vi "Old_XLIN1.7-2048SQ TE0_Host.vi"() -> ()   [LabVIEW 2018]
uses:
  <instrlib>/niDCPower/nidcpower.llb/niDCPower Measurement Type.ctl
  <instrlib>/niDMM/nidmm.llb/niDMM Function.ctl
  <instrlib>/niDMM/nidmm.llb/niDMM Resolution in Digits.ctl
  <vilib>/FPGAPlugInAG/PXI-7953R/niLvFpga_Open_PXI-7953R.vi
  <vilib>/rvi/interface/common/dynamic/niFpgaDynamicAddResources.vi
  <vilib>/FPGAPlugInAG/Dynamic/niLvFpga_Reset_Dynamic.vi
  <vilib>/FPGAPlugInAG/Dynamic/niLvFpga_Run_Dynamic.vi
  <vilib>/Utility/error.llb/Error Cluster From Error Code.vi
  <vilib>/rvi/errors/niLvFpgaAdjustHostInterfaceError.vi
  <instrlib>/niDMM/nidmm.llb/niDMM Configure Measurement Digits.vi
  <vilib>/FPGAPlugInAG/Dynamic/niLvFpga_Close_Dynamic.vi
  <vilib>/rvi/interface/nirviOpenFPGA/nirviOpenFPGA.xnode
  FPGA Bitfiles/XLIN1.7-2048SQTE_FPGATarget_XLIN1.7-2048SQTE_AuhCl0rpp4A.lvbitx
  <vilib>/rvi/interface/nirviMethod/nirviMethod.xnode
  <vilib>/rvi/interface/nirviReadWriteControl/nirviReadWriteControl.xnode
  <vilib>/rvi/interface/nirviCloseFPGA/nirviCloseFPGA.xnode
  NiFpgaLv.dll
  <vilib>/rvi/interface/Simulation/niFpgaSimulationCallBeginRW.vi
  <vilib>/FPGAPlugInAG/Dynamic/niLvFpga_ReadFifo_Dynamic.vi
  <vilib>/rvi/errors/niLvFpgaMergeErrorWithErrorCode.vi
panel:
  in  "Tab Control":T1(tab)
  in  "Clean Table":bool caption="Clear"
  in  "VDDD ON":bool
  out "VDDD_char":dbl(graph)=8.200132019086688e-05
  in  "VDDD, V":dbl=3.3000000000000003 caption="voltage level" min=0.0 max=6.0 format="%_6p"
  out "VDDD_cur, A":dbl=8.200132019086688e-05 caption="measurement" format="%_6g"
  in  "VDDD_curlim, A":dbl=0.5 caption="current limit" min=0.01 max=1.0 format="%_6p"
  in  "VDDD_selcur, A":dbl=0.49 caption="current limit" format="%_6p"
  out "VDDA_warning":bool caption="VCC_warning"
  out "VDDD_counter":u32 caption="VCC_counter"
  in  "VDDA ON":bool
  out "VDDA_char":dbl(graph)=9.464711192498274e-07
  in  "VDDA, V":dbl=3.3 caption="voltage level" min=0.0 max=20.0 format="%_6p"
  out "VDDA_cur, A":dbl=9.464711192498274e-07 caption="measurement" format="%_6g"
  in  "VDDA_curlim, A":dbl=0.5 caption="current limit" min=0.01 max=1.0 format="%_6p"
  in  "VDDA_selcur, A":dbl=0.49 caption="current limit" format="%_6p"
  out "VDDD_warning":bool caption="VCC_warning"
  out "VDDA_counter":u32 caption="VCC_counter"
  in  "Logs Path":path=path "D:/NI LabVIEW/21.056 XLIN1.7-2048SQ TE0/LOGS"
  in  "DC POWER 1":refnum<k15>="PXI1Slot2_2" caption="VСС_+5"
  in  "DC POWER 2":refnum<k15>="PXI1Slot3_3" caption="VСС_+5"
  in  "FPGA":tag="RIO0"
  in  "LED IR ON":bool
  out "LED IR_char":dbl(graph)=1.4003158139382402e-06
  in  "LED IR, V":dbl=-1.3000000000000003 caption="voltage level" min=-20.0 max=0.0 format="%_6p"
  out "LED IR_cur, A":dbl=1.4003158139382402e-06 caption="measurement" format="%_6g"
  in  "LED IR_curlim, A":dbl=0.4 caption="current limit" min=0.01 max=1.0 format="%_6p"
  out "Образец №":string
  in  "STOP":bool
  out "FIFOIsDone":bool
  out "FirmwareIsDone":bool
  out "PreCaptureIsDone":bool
  out "Frame Is Done":bool
  in  "Save":bool
  in  "Темный(F)\nСветлый(T)":bool
  in  "Примечание":string
  in  "VDDA_Clear_SEL":bool caption="Clear"
  in  "VDDD_Clear_SEL":bool caption="Clear"
  in  "Capture":bool
  in  "SEL Poll Time":u32=1
  in  "Автомат":bool
  in  "Питание":bool
  in  "SIM_SEL":bool
  in  "Loop Capture":bool
  in  "NI DMM":refnum<k15>="PXI1Slot4"
  in  "Опросить DMM":bool caption="Опрос DMM"
  in  "U_AOS Table":string[][](table)=[["", "Voltage", "", ""], ["OutTop_n", "", "", ""], ["OutTop_p", "", "", ""], ["OutBot_p", "", "", ""], ["OutBot_n", "", "", ""], ["U_AOS_Top", "", "", ""], ["U_AOS_Bot", "", "", ""]] caption="Размах аналогового выхода"
  in  "RS":bool
  in  "Очистить ОС":bool caption="Clear"
  out "Счетчик ОС":u32
  in  "+0.5_Clear_SEL":bool caption="Clear"
  out "+6_counter":u32 caption="VCC_counter"
  out "+6_warning":bool caption="VCC_warning"
  in  "+6_selcur, A":dbl=0.49 caption="current limit" format="%_6p"
  in  "+6, A":dbl=0.5 caption="current limit" min=0.01 max=1.0 format="%_6p"
  out "+6_cur, A":dbl=0.00011627237241327378 caption="measurement" format="%_6g"
  in  "+6, V":dbl=6.0 caption="voltage level" min=0.0 max=6.0 format="%_6p"
  out "+6_char":dbl(graph)=0.00011627237241327378
  in  "+6 ON":bool
  in  "Этап прошивки":T2(ring)
  in  "Firmware":bool
  out "Command":u8[](array[numeric])
  out "Data":u8[](array[numeric])
  out "ArraySize":u8
  in  "XLIN Rise Time":u32=500
  out "ADC Configuration":bool
  in  "Frame Poll Time":u32=500
  out "+0.5_counter":u32 caption="VCC_counter"
  out "+0.5_warning":bool caption="VCC_warning"
  in  "+0.5_selcur, A":dbl=0.09 caption="current limit" format="%_6p"
  in  "+0.5_curlim, A":dbl=0.1 caption="current limit" min=0.01 max=1.0 format="%_6p"
  out "+0.5_cur, A":dbl=-6.586231837824974e-06 caption="measurement" format="%_6g"
  in  "+0.5, V":dbl=0.5 caption="voltage level" min=0.0 max=20.0 format="%_6p"
  out "+0,5_char":dbl(graph)=-6.586231837824974e-06
  in  "+0.5 ON":bool
  in  "ОС":bool
  out "Счетчик ФС":u32
  in  "Очистить ФС":bool caption="Clear"
  in  "Минус ОС":bool
  in  "Плюс ОС":bool
  in  "Минус ФС":bool
  in  "Плюс ФС":bool
  in  "ADC Rise Time":u32=500
  out "АЦП прошит!":bool
  in  "ФС":bool
  in  "Задержка прошивки":u32=1
  out "Power VDDD+VDDA, mW":string
  in  "+6_Clear_SEL":bool caption="Clear"
  out "Image":T3(plugin-control)
  in  "Top":bool=TRUE
  in  "Bot":bool=TRUE
  in  "Capture Format":enum16{"Top / Bot", "Top & Bot"}(ring)
  in  "Frame Exposure, ms":u32=100
  in  "Delay Between Top&Bot":u32=5
  out "Configuration":bool[](array[boolean])
  in  "3CH/1CH":enum16{"3CH", "1CH"}(ring)=enum."1CH"
  in  "2/4 V":enum16{"2V", "4V"}(ring)=enum."4V"
  in  "+/- GREEN":enum16{"-", "+"}(ring)=enum."+"
  in  "Смещение, до 300_GREEN":dbl
  in  "+/- RED":enum16{"-", "+"}(ring)=enum."+"
  in  "Смещение, до 300_RED":dbl
  in  "+/- BLUE":enum16{"-", "+"}(ring)=enum."+"
  in  "Смещение, до 300_BLUE":dbl
  in  "Усиление (до 6)_GREEN":u8=1
  in  "Усиление (до 6)_BLUE":u8=1
  in  "Усиление (до 6)_RED":u8=1
  in  "Какой канал?":enum16{"GREEN", "RED", "BLUE"}(ring)=enum."BLUE"
  in  "Прошить АЦП":bool
  in  "ADC Register Map":T4(ring)
  out "MUX":bool[](array[boolean])
  in  "TopVIN":enum16{"GREEN", "RED", "BLUE"}(ring)=enum."RED"
  in  "Bot VIN":enum16{"GREEN", "RED", "BLUE"}(ring)
  in  "7..0(F)/0..7(T)":bool
  in  "F(F)/R(T)_CmAD":bool
  in  "F(F)/R(T)_FIFO":bool=TRUE
  in  "Command CS":u8[](array[numeric])=[8, 4, 2, 2, 2, 2, 2, 2, 2, 2, 2, 2, 2, 2, 2, 2, 2, 2, 2, 2, 2, 2, 2, 2, 2, 2, 2, 2, 2, 2, 2, 2, 2, 8, 4, 1, 1, 1, 1, 1, 1, 1, 1, 1, 0]
  in  "Data CSTop":u8[](array[numeric])=[0, 9, 12, 11, 0, 6, 0, 2, 11, 0, 8, 0, 0, 0, 0, 9, 1, 3, 3, 7, 15, 15, 5, 15, 0, 1, 15, 15, 5, 8, 5, 2, 3, 0, 8, 2, 3, 3, 3, 3, 3, 3, 3, 2, 0]
  in  "Data CSBot":u8[](array[numeric])=[0, 9, 8, 11, 0, 6, 0, 2, 11, 0, 8, 0, 0, 0, 0, 9, 1, 3, 11, 7, 15, 15, 5, 15, 0, 1, 15, 15, 5, 8, 5, 2, 3, 0, 8, 2, 3, 3, 3, 3, 3, 3, 3, 2, 0]
  in  "Command Reset":u8[](array[numeric])=[8, 4, 2, 2, 2, 2, 9, 0]
  in  "Data Reset":u8[](array[numeric])=[0, 0, 0, 5, 0, 0, 0, 0]
  in  "Command Hold":u8[](array[numeric])=[8, 4, 2, 2, 2, 2, 9, 2, 2, 2, 2, 2, 0, 0, 0, 0, 0, 8, 4, 2, 2, 2, 2, 9, 2, 2, 2, 2, 9, 2, 2, 2, 2, 9, 2, 2, 2, 2, 9, 2, 2, 2, 2, 9, 2, 2, 2, 2, 9, 0, 0]
  in  "Data Hold":u8[](array[numeric])=[0, 0, 0, 1, 1, 0, 0, 0, 5, 1, 0, 0, 0, 0, 0, 0, 0, 0, 0, 0, 3, 1, 0, 0, 1, 5, 1, 0, 0, 1, 3, 1, 0, 0, 1, 3, 1, 0, 0, 1, 11, 1, 11, 0, 1, 11, 1, 3, 0, 0, 0]
  in  "Command Sample Start":u8[](array[numeric])=[8, 4, 2, 2, 2, 2, 9, 2, 2, 2, 2, 2, 2, 1, 1, 1, 1, 1, 1, 0]
  in  "Data Sample Start":u8[](array[numeric])=[0, 0, 1, 11, 1, 0, 0, 0, 0, 6, 0, 0, 15, 0, 1, 3, 5, 13, 13, 0]
  in  "Command Sample End":u8[](array[numeric])=[8, 4, 2, 0, 0]
  in  "Data Sample End":u8[](array[numeric])=[0, 5, 1, 0, 0]
  in  "Supply Select":u8(ring) items=["Local", "External"]
  in  "1032 pixels":u16=1032
  in  "NumberOfAddFIFO":u16=2064
  in  "Falling CLK_1 = 1":u8=1
  in  "Rising CLK_1 = 0":u8
  in  "Rising CLK_2 = 1":u8=1
  in  "Falling CLK_2 = 2":u8=2
  in  "Rising CLK_3 = 1":u8=1
  in  "Falling CLK_3 = 1":u8=1
  in  "Falling CLK_4 = 3":u8=3
  in  "Rising CLK_4 = 2":u8=2
  in  "Rising CLK_5 = 2":u8=2
  in  "Falling CLK_5 = 2":u8=2
  in  "Falling CLK_6 = 2":u8=2
  in  "Rising CLK_6 = 2":u8=1
  in  "Falling CLK_7 = 1":u8=1
  in  "Rising CLK_7 = 1":u8=1
  in  "Counter R&F CLK_1 = 7":u8=7
  in  "Counter R&F CLK_2 = 4":u8=4
  in  "R ADCCLK = 5":u16=5
  in  "R MCLK = 2":u16=2
  in  "Counter R CLK = 2":u8=2
  out "FIFOCounter":u16
  out "SEL output file refnum":refnum<file>
  out "Power OFF":bool
  in  "Считать SIM SEL":bool
  out "Ready Status":bool
  out "NI DMM Real Voltage":dbl format="%.15f"
  out "NI DMM output file":refnum<file>
  out "NI DMM Voltage":dbl caption="Voltage" format="%_6g"
  out "NI DMM Voltage Char":dbl(graph)=0.6705812438667635
  in  "NI DMM units":string(combo)="1" caption="Units"
  in  "NI DMM Voltage Range":string(combo)="10" caption="Range"
  in  "NI DMM Poll Time":u32=100 caption="DMM Poll Time"
  in  "NI DMM Samples":i32=10
  out "Voltage Sum":dbl format="%.15f"
  in  "U_AOS":dbl[](array[numeric])=[0.0, 0.0, 0.0, 0.0, 0.0, 0.0]
  in  "PreCapture":bool
  in  "Start":bool
  out "SEL_warning":bool caption="SEL"
  out "Test Model Log Path":path
  out "Bot Pixel":bool[](array[boolean])
  out "Top Pixel":bool[](array[boolean])
  out "FrameDataFromTop":u8[](array[numeric])
  out "FrameDataFromBot":u8[](array[numeric])
  out "LineOfBot":u16[](array[numeric])
  out "LineOfTop":u16[](array[numeric])
  in  "WatchDogFIFOTime":u32=1000
  out "FIFOTime":u32
  out "Full Line":u16[](array[numeric])
  # "CH0 VDDD\nCH1 VDDA\nCH2 LED IR"
  # "CH0 +6\nCH1 +0,5"
  # "DC1 CH0"
  # "DC1 CH1"
  # "DC2 CH1"
  # "DC2 CH2"
  # "DC2 CH2"
  # "Добавить 8й элемент"
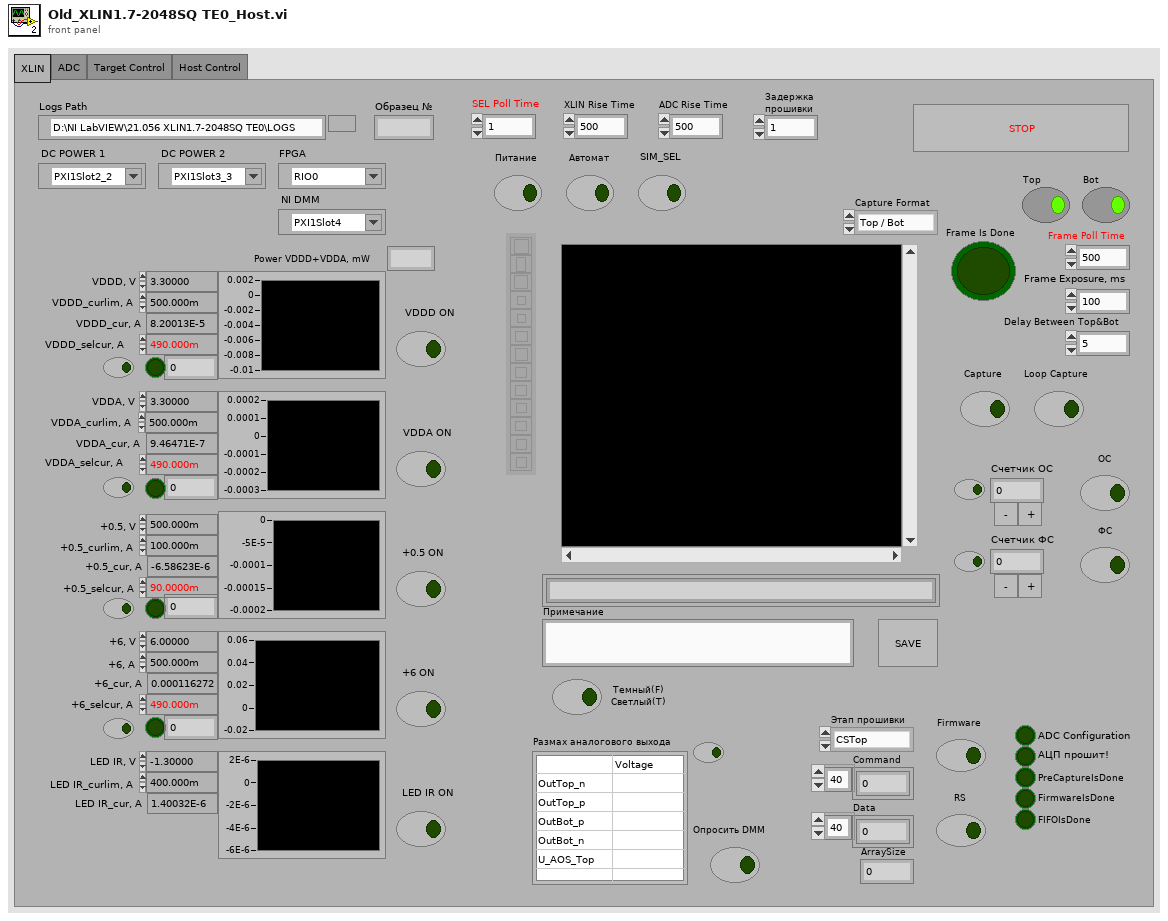
[diagram p1: front panel]
types:
  T1 = enum32{"XLIN", "ADC", "Target Control", "Host Control"}
  T2 = enum16{"CSTop", "CSBot", "Reset", "Hold", "Sample Start", "Sample End"}
  T3 = typedef "IMAQ Image.ctl" = refnum<image>
  T4 = enum16{"Configuration", "MUX", "RED PGA", "GREEN PGA", "BLUE PGA", "RED OFF", "GREEN OFF", "BLUE OFF"}
  T5 = enum16{"open", "replace", "create", "open or create", "replace or create", "replace or create with confirmation"}
  T6 = typedef "Image Type" = u32
  T7 = typedef "niDMM Function.ctl" = enum16{"DC Volts", "AC Volts", "DC Current", "AC Current", "2-wire Resistance", "4-wire Resistance", "Diode", "Frequency", "Period", "AC Volts DC Coupled", "Capacitance", "Inductance", "Temperature"}
  T8 = typedef "niDMM Resolution in Digits.ctl" = dbl
  T9 = typedef "niDCPower Measurement Type.ctl" = i32
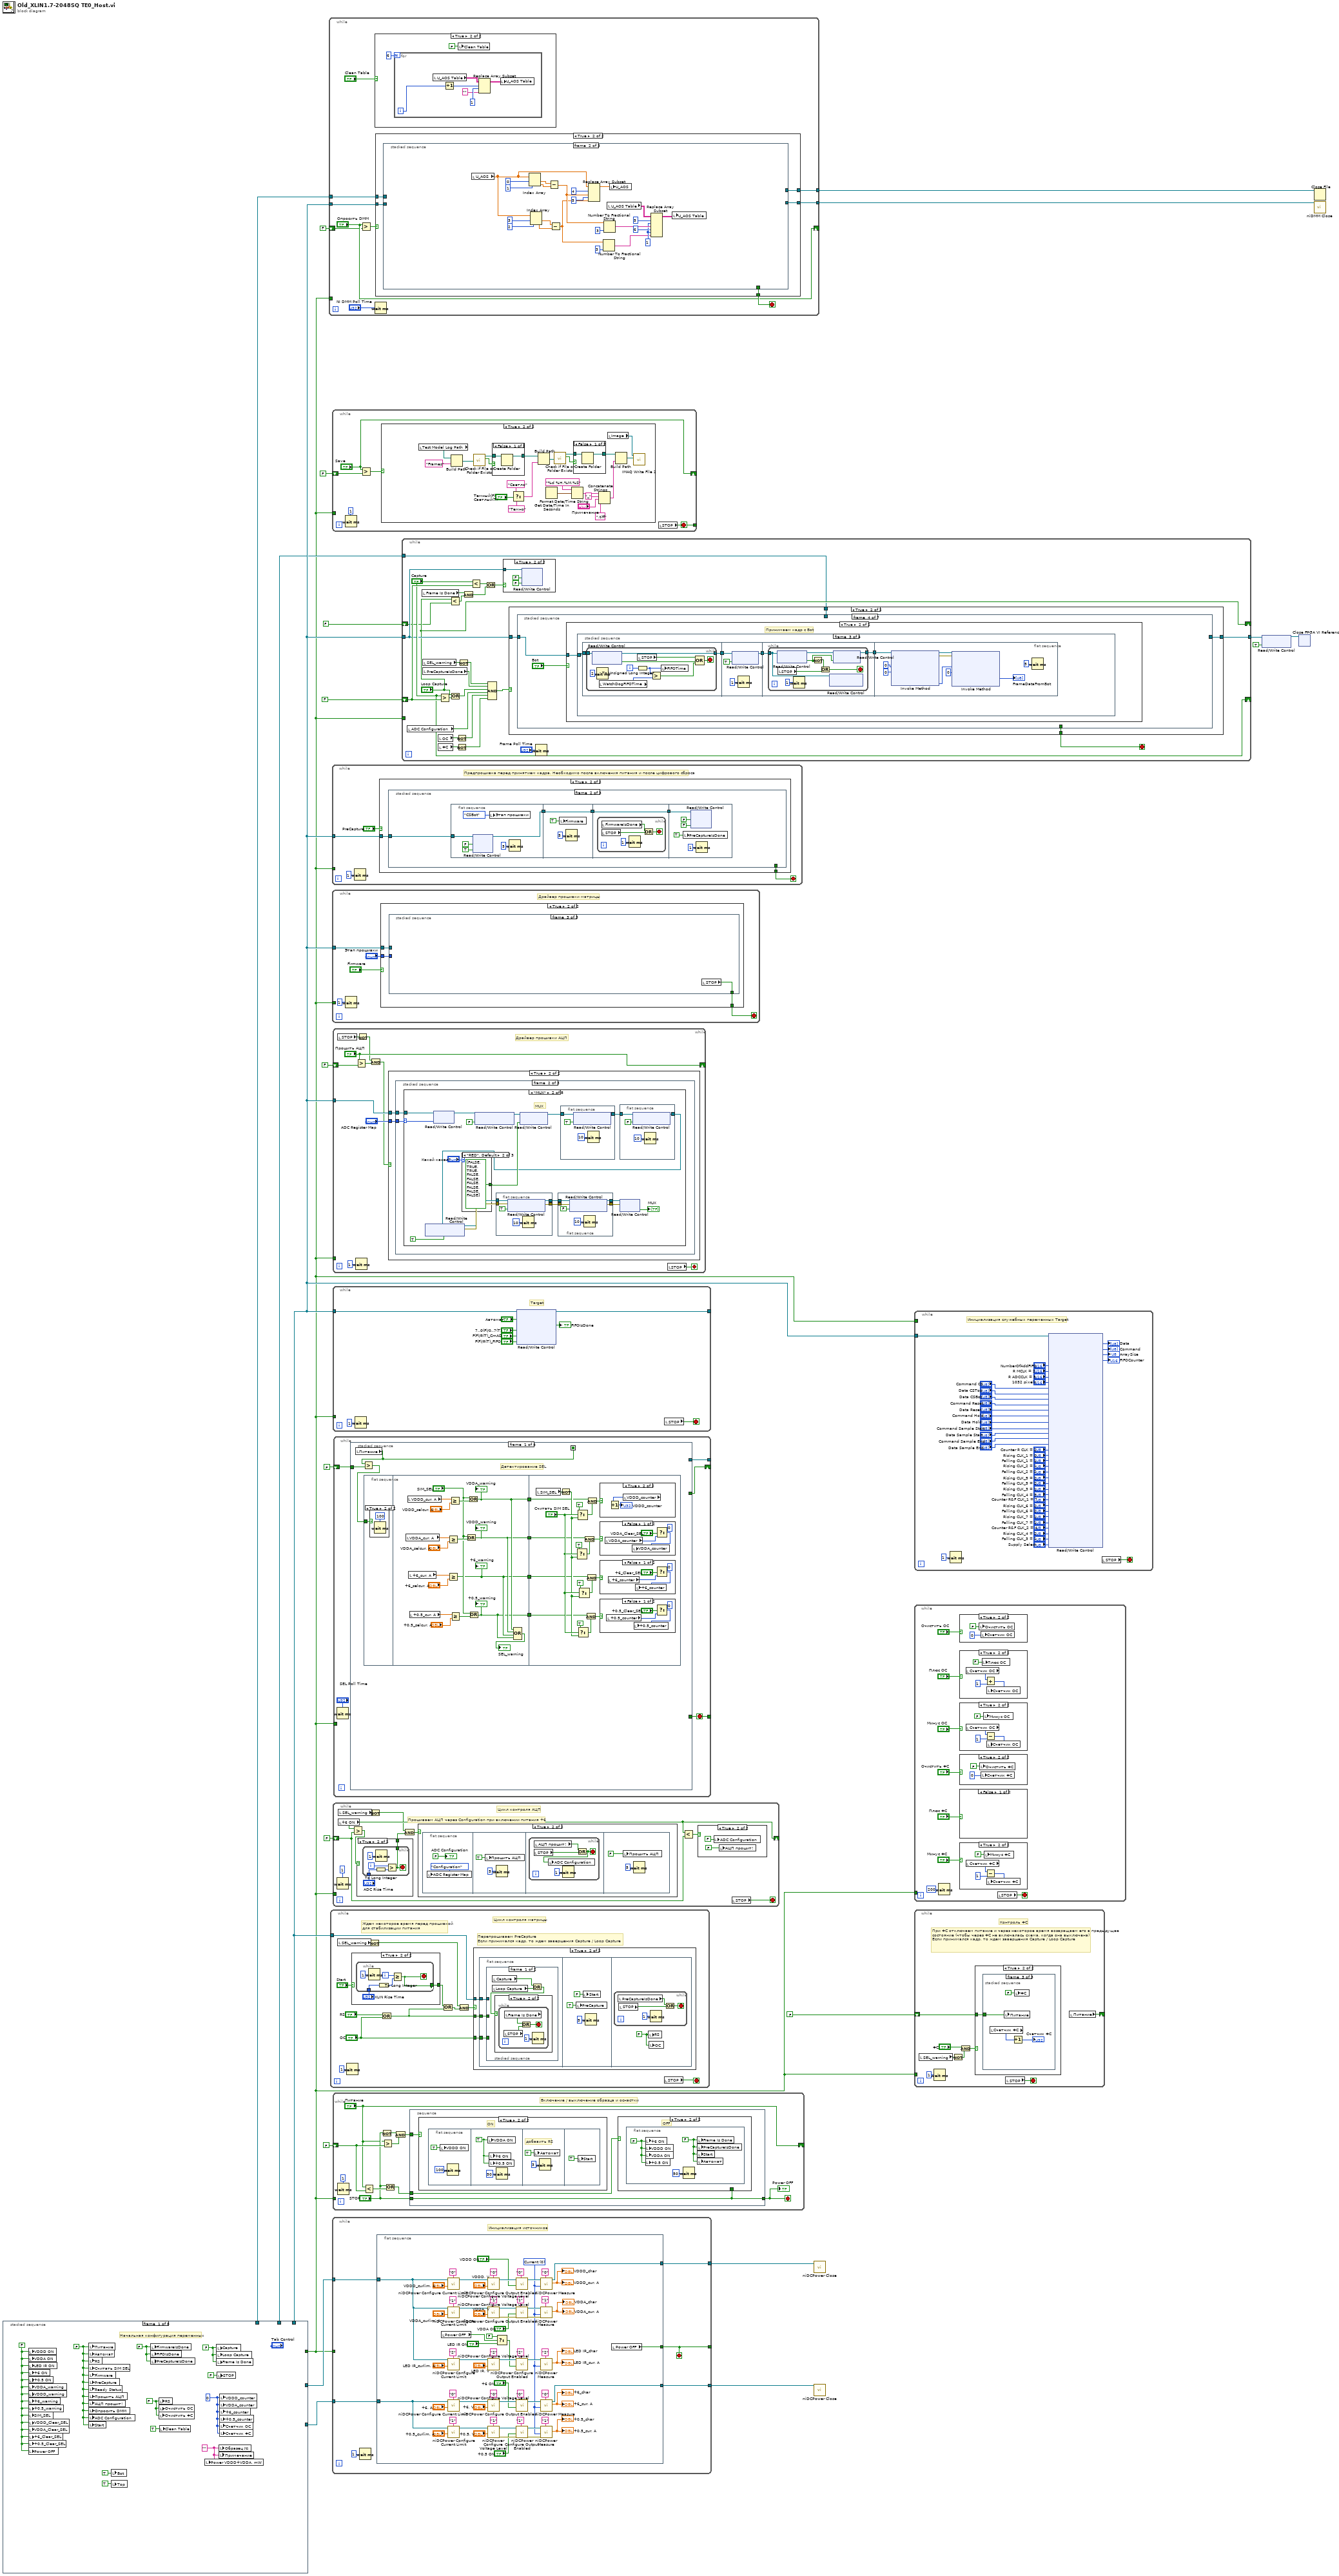
[diagram p0: block diagram]
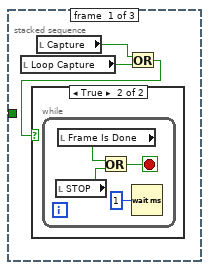
[diagram p3: hidden frame]
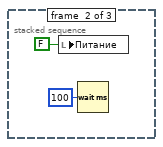
[diagram p5: hidden frame]
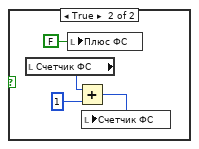
[diagram p7: hidden frame]
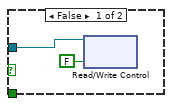
[diagram p16: hidden frame]
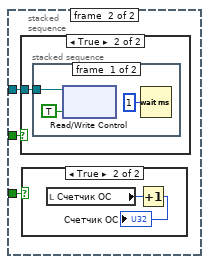
[diagram p18: hidden frame]
diagram:
  n1 = stacked-sequence {
    tunnel: [_ _ _ _ _ _ w138 _] -> w20
    tunnel: [_ _ _ _ _ _ w137 _] -> w19
    tunnel: [_ w34 _ _ _ _ _ _] -> w4
    tunnel: [_ _ _ _ _ w129 _ _] -> w9
    tunnel: [_ _ _ _ _ _ _ w149] -> w3
    tunnel: [_ _ _ _ _ _ w135 _] -> w13
    frame #0 {
      w26 = FALSE ("RS")
      w27 = u32 0 ("VDDD_counter")
      w25 = "" ("Образец №")
      w32 = FALSE ("Питание")
      w31 = FALSE ("Питание")
      w28 = FALSE ("Питание")
      w33 = FALSE ("VDDD ON")
      # "Начальная конфигурация переменных"
      n2 = local write "VDDD ON"(w33) -> ()
      n3 = local write "VDDA ON"(w33) -> ()
      n4 = local write "LED IR ON"(w33) -> ()
      n5 = local write "+6 ON"(w33) -> ()
      n6 = local write "+0.5 ON"(w33) -> ()
      n7 = local write "VDDA_warning"(w33) -> ()
      n8 = local write "VDDD_warning"(w33) -> ()
      n9 = local write "+6_warning"(w33) -> ()
      n10 = local write "+0.5_warning"(w33) -> ()
      n11 = local write "SIM_SEL"(w33) -> ()
      n12 = local write "VDDD_Clear_SEL"(w33) -> ()
      n13 = local write "VDDA_Clear_SEL"(w33) -> ()
      n14 = local write "+6_Clear_SEL"(w33) -> ()
      n15 = local write "+0.5_Clear_SEL"(w33) -> ()
      n16 = local write "Power OFF"(w33) -> ()
      n17 = local write "Питание"(w28) -> ()
      n18 = local write "Автомат"(w28) -> ()
      n19 = local write "RS"(w28) -> ()
      n20 = local write "Считать SIM SEL"(w28) -> ()
      n21 = local write "Firmware"(w28) -> ()
      n22 = local write "PreCapture"(w28) -> ()
      n23 = local write "Ready Status"(w28) -> ()
      n24 = local write "Прошить АЦП"(w28) -> ()
      n25 = local write "АЦП прошит!"(w28) -> ()
      n26 = local write "Опросить DMM"(w28) -> ()
      n27 = local write "ADC Configuration"(w28) -> ()
      n28 = local write "Start"(w28) -> ()
      n29 = local write "Bot"(TRUE ("Bot")) -> ()
      n30 = local write "Top"(TRUE ("Top")) -> ()
      n31 = local write "FirmwareIsDone"(w31) -> ()
      n32 = local write "FIFOIsDone"(w31) -> ()
      n33 = local write "PreCaptureIsDone"(w31) -> ()
      n34 = local write "RS"(w26) -> ()
      n35 = local write "Очистить ОС"(w26) -> ()
      n36 = local write "Очистить ФС"(w26) -> ()
      n37 = local write "Clean Table"(TRUE ("Clean Table")) -> ()
      n38 = local write "Power VDDD+VDDA, mW"(w25) -> ()
      n39 = local write "Capture"(w32) -> ()
      n40 = local write "Loop Capture"(w32) -> ()
      n41 = local write "Frame Is Done"(w32) -> ()
      n42 = local write "STOP"(FALSE ("STOP")) -> ()
      n43 = local write "Образец №"(w25) -> ()
      n44 = local write "Примечание"(w25) -> ()
      n45 = local write "VDDD_counter"(w27) -> ()
      n46 = local write "VDDA_counter"(w27) -> ()
      n47 = local write "+6_counter"(w27) -> ()
      n48 = local write "+0.5_counter"(w27) -> ()
      n49 = local write "Счетчик ОС"(w27) -> ()
      n50 = local write "Счетчик ФС"(w27) -> ()
    }
    frame #1 {
      w35 = T6 7 items=["Grayscale (U8)", "Grayscale (I16)", "Grayscale (SGL)", "Complex (CSG)", "RGB (U32)", "HSL (U32)", "RGB (U64)", "Grayscale (U16)"] ("Image Type")
      n51 = call "IMAQ Create"("Image Name"="XLIN1.7-2048SQ TE0", "Image Type"=w35) -> ("New Image"=w34:T3)  [unwired: 3 in, 1 out]
    }
    frame #2 {
      n52 = call "XLIN1.7-2048SQ TE0_Begin.vi"() -> ("Текущий Образец №"=→"Образец №":string)
    }
    frame #3 {
      w40 = "\t"
      # "Инициализация файла"
      n53 = local read "Образец №"() -> (w70:string)
      n54 = Build Path(base path="Logs Path", name or relative path=w70) -> (appended path=w65:path)
      n55 = call <vilib>:"Check if File or Folder Exists.vi"("path"=w65) -> ("file or folder exists?"=w66:bool, "dup path"=w67:path)  [unwired: 8 in, 1 out]
      "Test Model Log Path" <- w67
      n56 = case shown="False" w66 {
        tunnel: w67 -> [w86 w87]
        tunnel: [w85 w87] -> w64
        frame False {
          n57 = Create Folder(path (use dialog)=w86) -> (created path=w85:path)  [unwired: 2 in, 2 out]
        }
        frame True {
        }
      }
      n58 = Build Path(base path=w64, name or relative path="SEL") -> (appended path=w63:path)
      n59 = Get Date/Time In Seconds() -> (seconds since 1Jan1904=w81:timestamp)
      n60 = call <vilib>:"Check if File or Folder Exists.vi"("path"=w63) -> ("file or folder exists?"=w84:bool, "dup path"=w83:path)  [unwired: 8 in, 1 out]
      n61 = Format Date/Time String(time format string (%c)="SEL 1 %d %m %y %H.%M.%S", seconds (now)=w81) -> (date/time string=w80:string)  [unwired: 1 in]
      n62 = case shown="False" w84 {
        tunnel: w83 -> [w89 w90]
        tunnel: [w88 w90] -> w82
        frame False {
          n63 = Create Folder(path (use dialog)=w89) -> (created path=w88:path)  [unwired: 2 in, 2 out]
        }
        frame True {
        }
      }
      n64 = Concatenate Strings(w80, ".xls" ("string")) -> (w78:string)
      n65 = Build Path(base path=w82, name or relative path=w78) -> (appended path=w75:path)
      n66 = Open/Create/Replace File(file path (use dialog)=w75, operation (0:open)=T5."open or create", access (0:read/write)=enum16{"read/write", "read-only", "write-only"}."read/write") -> (refnum out=w74:refnum<file>)  [unwired: 3 in, 2 out]
      n67 = Set File Position(refnum=w74, from (0:start)=enum16{"start", "end", "current"}."end") -> (refnum out=w72:refnum<file>)  [unwired: 2 in, 1 out]
      n68 = Format Into String(initial string=w72, "Time" ("string"), w40, "VDDD, V" ("string"), w40, "VDDD_cur, A" ("string"), w40, "VDDD_SEL" ("string"), w40, "!!!" ("string"), w40, "VDDA, V" ("string"), w40, "VDDA_cur, A" ("string"), w40, "VDDA_SEL" ("string"), w40, "!!!" ("string"), w40, "+6, V" ("string"), w40, "+6_cur, A" ("string"), w40, "+6_SEL" ("string"), w40, "!!!" ("string"), w40, "+0,5, V" ("string"), w40, "+0,5_cur, A" ("string"), w40, "+0.5_SEL" ("string"), w40, "!!!" ("string"), w40, "LED IR, V" ("string"), w40, "LED IR_cur, A" ("string"), w40, "Power, mW" ("string"), w40, "ОС" ("string"), w40, "ФС" ("string"), "\r\n") -> (resulting string=→"SEL output file refnum":refnum<file>)  [unwired: 2 in, 1 out]
    }
    frame #4 {
      w93 = "\t"
      n69 = local read "Logs Path"() -> (w105:path)
      n70 = local read "Образец №"() -> (w116:string)
      n71 = Build Path(base path=w105, name or relative path=w116) -> (appended path=w102:path)
      n72 = call <vilib>:"Check if File or Folder Exists.vi"("path"=w102) -> ("file or folder exists?"=w103:bool, "dup path"=w104:path)  [unwired: 8 in, 1 out]
      n73 = case shown="False" w103 {
        tunnel: w104 -> [w124 w125]
        tunnel: [w123 w125] -> w99
        frame False {
          n74 = Create Folder(path (use dialog)=w124) -> (created path=w123:path)  [unwired: 2 in, 2 out]
        }
        frame True {
        }
      }
      n75 = Build Path(base path=w99, name or relative path="DMM") -> (appended path=w100:path)
      n76 = Get Date/Time In Seconds() -> (seconds since 1Jan1904=w119:timestamp)
      n77 = call <vilib>:"Check if File or Folder Exists.vi"("path"=w100) -> ("file or folder exists?"=w122:bool, "dup path"=w121:path)  [unwired: 8 in, 1 out]
      n78 = Format Date/Time String(time format string (%c)="NI DMM 1 %d %m %y %H.%M.%S", seconds (now)=w119) -> (date/time string=w118:string)  [unwired: 1 in]
      n79 = case shown="False" w122 {
        tunnel: w121 -> [w127 w128]
        tunnel: [w126 w128] -> w120
        frame False {
          n80 = Create Folder(path (use dialog)=w127) -> (created path=w126:path)  [unwired: 2 in, 2 out]
        }
        frame True {
        }
      }
      n81 = Concatenate Strings(w118, ".xls" ("string")) -> (w117:string)
      n82 = Build Path(base path=w120, name or relative path=w117) -> (appended path=w113:path)
      n83 = Open/Create/Replace File(file path (use dialog)=w113, operation (0:open)=T5."open or create", access (0:read/write)=enum16{"read/write", "read-only", "write-only"}."read/write") -> (refnum out=w115:refnum<file>)  [unwired: 3 in, 2 out]
      n84 = Set File Position(refnum=w115, from (0:start)=enum16{"start", "end", "current"}."end") -> (refnum out=w114:refnum<file>)  [unwired: 2 in, 1 out]
      n85 = Format Into String(initial string=w114, "Time" ("string"), w93, "OutTop_n, V" ("string"), w93, "OutTop_p, V" ("string"), w93, "OutBot_p, V" ("string"), w93, "OutBot_n, V" ("string"), w93, "U_AOS Top, V" ("string"), w93, "U_AOS Bot, V" ("string"), "\r\n") -> (resulting string=→"NI DMM output file":refnum<file>)  [unwired: 2 in, 1 out]
    }
    frame #5 {
      # "Подключение FPGA"
      n86 = xnode "Open FPGA VI Reference"("resource name"="FPGA") -> ("FPGA VI Reference Out"=w133:refnum<k20>, "error out"=w131:errorcluster)  [unwired: 1 in]
      n87 = xnode "Invoke Method"("FPGA VI Reference In"=w133, "error in"=w131) -> ("FPGA VI Reference Out"=w130:refnum<k20>, "error out"=w132:errorcluster)
      n88 = xnode "Invoke Method"("FPGA VI Reference In"=w130, "error in"=w132) -> ("FPGA VI Reference Out"=w129:refnum<k20>)  [unwired: 1 in, 1 out]
    }
    frame #6 {
      n89 = call <instrlib>:"niDCPower Initialize.vi"("resource name"="DC POWER 1") -> ("error out"=w147:errorcluster, "instrument handle out"=w148:refnum<k15>)  [unwired: 3 in, 6 out]
      n90 = call <instrlib>:"niDCPower Initialize.vi"("resource name"="DC POWER 2") -> ("error out"=w142:errorcluster, "instrument handle out"=w143:refnum<k15>)  [unwired: 3 in, 6 out]
      n91 = call <instrlib>:"niDMM Initialize.vi"("Instrument Descriptor"="NI DMM") -> ("instrument handle out"=w135:refnum<k15>)  [unwired: 9 in, 1 out]
      n92 = call <instrlib>:"niDCPower Configure Voltage Level.vi"("error in (no error)"=w147, "voltage level"=0.0, "channel name"="0:2", "instrument handle"=w148) -> ("instrument handle out"=w138:refnum<k15>)  [unwired: 6 in, 1 out]
      n93 = call <instrlib>:"niDCPower Configure Voltage Level.vi"("error in (no error)"=w142, "voltage level"=0.0, "channel name"="0:2", "instrument handle"=w143) -> ("instrument handle out"=w137:refnum<k15>)  [unwired: 6 in, 1 out]
    }
    frame #7 {
      w149 = TRUE ("Boolean")
      "Ready Status" <- w149
    }
  }
  n94 = while {
    tunnel: w13 -> [w159]
    tunnel: [w158] -> w15
    tunnel: [w157] -> w14
    tunnel: w3 -> [_]
    tunnel: w9 -> [w154]
    shift-right: ["Опросить DMM"] -> _
    shift-left: FALSE ("Опрос DMM") -> [w151]
    stop <- w155 stop-if-true
    n95 = Greater?(x="Опросить DMM", y=w151) -> (0:w153:bool)
    n96 = Wait (ms)(milliseconds to wait="NI DMM Poll Time") -> ()  [unwired: 1 out]
    n97 = case shown="True" "Clean Table" {
      frame False {
      }
      frame True {
        n98 = for {
          N: 6 -> [_]
          i -> [w166]
          n99 = local read "U_AOS Table"() -> (w165:string[][])
          n100 = Increment(x=w166) -> (x+1=w167:i32)
          n101 = Replace Array Subset(array=w165, new element="" ("new element/subarray"), index (row)=w167, index (col)=1 ("disabled index (col)")) -> (w162:string[][])
          n102 = local write "U_AOS Table"(w162) -> ()
        }
        n103 = local write "Clean Table"(FALSE ("Clean Table")) -> ()
      }
    }
    n104 = case shown="True" w153 {
      tunnel: w159 -> [w170 w175]
      tunnel: [w168 w172] -> w158
      tunnel: [w170 w174] -> w157
      tunnel: [w169 w171] -> w155
      tunnel: w154 -> [_ w173]
      frame False {
        n105 = local read "STOP"() -> (w169:bool)
        n106 = local read "NI DMM output file"() -> (w168:refnum<file>)
      }
      frame True {
        n107 = stacked-sequence {
          tunnel: w175 -> [w179 _ _]
          tunnel: [w178 _ _] -> w174
          tunnel: w173 -> [w176 _ w256]
          tunnel: [_ _ w258] -> w172
          tunnel: [_ _ w257] -> w171
          frame #0 {
            n108 = for {
              N: 4 -> [_]
              shift-right: [w182] -> w178
              shift-left: w179 -> [w183]
              tunnel: w176 -> [w180]
              i -> [w181]
              n109 = stacked-sequence {
                tunnel: w183 -> [_ w195 _]
                tunnel: [_ w194 _] -> w182
                tunnel: w181 -> [w191 _ w220]
                tunnel: w180 -> [w184 _ _]
                frame #0 {
                  n110 = Number To Boolean Array(number=w191) -> (Boolean array=w190:bool[])
                  n111 = Index Array(array=w190, index=1) -> (element=w186:bool)
                  n112 = Index Array(array=w190, index=0) -> (element=w187:bool)
                  n113 = Wait (ms)(milliseconds to wait=u32 1) -> ()  [unwired: 1 out]
                  n114 = xnode "Read/Write Control"("FPGA VI Reference In"=w184, "IN2"=w187, "IN1"=w186) -> ()  [unwired: 1 in, 2 out]
                }
                frame #1 {
                  n115 = for {
                    N: "NI DMM Samples" -> [_]
                    shift-right: [w199] -> w194
                    shift-left: w195 -> [w200]
                    shift-right: [w196] -> _
                    shift-left: 0.0 ("Measurement") -> [w198]
                    n116 = flat-sequence {
                      tunnel: [w207] -> w203
                      tunnel: w200 -> [w206]
                      tunnel: w203 -> [w211]
                      tunnel: [w214] -> w202
                      tunnel: [w210] -> w201
                      tunnel: w202 -> [w219]
                      tunnel: [w219] -> w199
                      tunnel: w201 -> [w217]
                      tunnel: w198 -> [w218]
                      tunnel: [w216] -> w196
                      frame #0 {
                        w204 = T8 6.5 items=["3 1/2"=3.5, "4 1/2"=4.5, "5 1/2"=5.5, "6 1/2"=6.5, "7 1/2"=7.5] ("Resolution in Digits")
                        n117 = Fract/Exp String To Number(string="NI DMM Voltage Range") -> (number=w208:dbl)  [unwired: 3 in, 1 out]
                        n118 = call-poly <instrlib>:"niDMM Config Measurement.vi"("Range"=w208, "Resolution in Digits"=w204, "Function"=niDMM_Function."DC Volts" ("Measurement Type"), "instrument handle"=w206) -> ("instrument handle out"=w207:refnum<k15>)  [unwired: 6 in, 1 out]
                      }
                      frame #1 {
                        n119 = call <instrlib>:"niDMM Read.vi"("instrument handle"=w211) -> ("Measurement"=w210:dbl, "instrument handle out"=w214:refnum<k15>)  [unwired: 8 in, 1 out]
                        "NI DMM Real Voltage" <- w210
                        n120 = Fract/Exp String To Number(string="NI DMM units") -> (number=w212:dbl)  [unwired: 3 in, 1 out]
                        n121 = Multiply(x=w212, y=w210) -> (x*y=→"NI DMM Voltage" →"NI DMM Voltage Char":dbl)
                      }
                      frame #2 {
                        n122 = Add(x=w217, y=w218) -> (x+y=w216:dbl)
                        "Voltage Sum" <- w216
                      }
                    }
                    n123 = Wait (ms)(milliseconds to wait=u32 1) -> ()  [unwired: 1 out]
                  }
                }
                frame #2 {
                  n124 = local read "NI DMM Samples"() -> (w227:i32)
                  n125 = local read "Voltage Sum"() -> (w232:dbl)
                  n126 = Increment(x=w220) -> (x+1=w221:i32)
                  n127 = To Double Precision Float(number=w227) -> (double precision float=w228:dbl)
                  n128 = Divide(x=w232, y=w228) -> (x/y=w222:dbl)
                  n129 = Number To Fractional String(number=w222, precision (6)=3) -> (F-format string=w225:string)  [unwired: 2 in]
                  n130 = Replace Array Subset(array="U_AOS", new element=w222, index=w220) -> (w223:dbl[])
                  n131 = local write "U_AOS"(w223) -> ()
                  n132 = Replace Array Subset(array="U_AOS Table", new element=w225, index (row)=w221, index (col)=1 ("disabled index (col)")) -> (w230:string[][])
                  n133 = local write "U_AOS Table"(w230) -> ()
                }
              }
            }
          }
          frame #1 {
            w243 = 1 ("disabled index (col)")
            n134 = local read "U_AOS"() -> (w251:dbl[])
            n135 = Index Array(array=w251, index #1=0 ("disabled index (row)"), index #2=1 ("index (row)")) -> (element #1=w255:dbl, element #2=w254:dbl)
            n136 = Index Array(array=w251, index #1=3 ("disabled index (row)"), index #2=2 ("index (row)")) -> (element #1=w253:dbl, element #2=w252:dbl)
            n137 = Subtract(x=w255, y=w254) -> (x-y=w247:dbl)
            n138 = Subtract(x=w253, y=w252) -> (x-y=w246:dbl)
            n139 = Replace Array Subset(array=w251, new element #1=w247, index #1=4 ("index (row)"), new element #2=w246, index #2=5 ("disabled index (row)")) -> (w250:dbl[])
            n140 = Number To Fractional String(number=w246, precision (6)=i16 3) -> (F-format string=w235:string)  [unwired: 2 in]
            n141 = Number To Fractional String(number=w247, precision (6)=i16 3) -> (F-format string=w245:string)  [unwired: 2 in]
            n142 = local read "U_AOS Table"() -> (w249:string[][])
            n143 = local write "U_AOS"(w250) -> ()
            n144 = Replace Array Subset(array=w249, new element #1=w245, index (row) #1=5 ("index (row)"), index (col) #1=w243, new element #2=w235, index (row) #2=6 ("disabled index (row)"), index (col) #2=w243) -> (w248:string[][])
            n145 = local write "U_AOS Table"(w248) -> ()
          }
          frame #2 {
            n146 = flat-sequence {
              tunnel: w261 -> [w267]
              tunnel: [w266] -> w260
              tunnel: w256 -> [w262]
              tunnel: w260 -> [w270]
              tunnel: [w269] -> w259
              tunnel: w259 -> [w282]
              tunnel: [w281] -> w258
              frame #0 {
                n147 = Format Date/Time String(time format string (%c)="%H:%M:%S:%3u") -> (date/time string=w265:string)  [unwired: 2 in]
                n148 = xnode "Read/Write Control"("FPGA VI Reference In"=w262, "IN2"=FALSE ("IN1"), "IN1"=FALSE ("IN2")) -> ()  [unwired: 1 in, 2 out]
                n149 = Format Into String(initial string=w267, w265) -> (resulting string=w266:refnum<file>)  [unwired: 2 in, 1 out]
              }
              frame #1 {
                n150 = for {
                  N: 6 -> [_]
                  tunnel: w270 -> [w276]
                  tunnel: [w275] -> w269
                  i -> [w278]
                  n151 = local read "U_AOS"() -> (w280:dbl[])
                  n152 = Index Array(array=w280, index=w278) -> (element=w279:dbl)
                  n153 = Number To Fractional String(number=w279, precision (6)=i16 15) -> (F-format string=w274:string)  [unwired: 2 in]
                  n154 = Concatenate Strings("\t", w274) -> (w277:string)
                  n155 = Format Into String(initial string=w276, w277) -> (resulting string=w275:refnum<file>)  [unwired: 2 in, 1 out]
                }
              }
              frame #2 {
                n156 = Format Into String(initial string=w282, "\r\n") -> (resulting string=w281:refnum<file>)  [unwired: 2 in, 1 out]
              }
            }
            n157 = local read "NI DMM output file"() -> (w261:refnum<file>)
            n158 = local read "STOP"() -> (w257:bool)
          }
        }
      }
    }
  }
  n159 = while {
    tunnel: w9 -> [w293]
    stop <- w294 stop-if-true
    # "Перепрошиваем PreCapture\nЕсли принимался кадр, то ждем завершения Capture / Loop Capture"
    # "Ждем некоторое время перед прошивкой для стабилизации питания"
    # "Цикл контроля матрицы"
    n160 = local read "SEL_warning"() -> (w287:bool)
    n161 = Wait (ms)(milliseconds to wait=u32 1) -> ()  [unwired: 1 out]
    n162 = case shown="True" "Start" {
      selector: "Start" -> [w296 _]
      tunnel: [w296 w298] -> w291
      frame False {
      }
      frame True {
        n163 = while {
          tunnel: [w300] -> w298
          tunnel: "XLIN Rise Time" -> [w299]
          i -> [w302]
          stop <- w300 stop-if-true
          n164 = Wait (ms)(milliseconds to wait=u32 1) -> ()  [unwired: 1 out]
          n165 = To Long Integer(number=w299) -> (32bit integer=w303:i32)
          n166 = Greater Or Equal?(x=w302, y=w303) -> (x >= y?=w300:bool)
        }
      }
    }
    n167 = Not(x=w287) -> (.not. x?=w286:bool)
    n168 = Or(x="RS", y="ОС") -> (x .or. y?=w290:bool)
    n169 = Compound Arithmetic op=OR(w291, w290) -> (w285:bool)
    n170 = Compound Arithmetic op=AND(w286, w285) -> (w284:bool)
    n171 = case shown="True" w284 {
      tunnel: w293 -> [w305 w308]
      tunnel: w290 -> [_ w307]
      tunnel: "ОС" -> [_ w306]
      frame False {
        n172 = xnode "Read/Write Control"("FPGA VI Reference In"=w305, "RS"=FALSE) -> ()  [unwired: 1 in, 2 out]
      }
      frame True {
        n173 = flat-sequence {
          tunnel: w308 -> [w311]
          tunnel: w307 -> [w310]
          tunnel: w306 -> [w309]
          frame #0 {
            n174 = stacked-sequence {
              tunnel: w311 -> [_ w321]
              tunnel: w310 -> [_ w320]
              tunnel: w309 -> [_ w319]
              frame #0 {
                n175 = local read "Loop Capture"() -> (w313:bool)
                n176 = local read "Capture"() -> (w314:bool)
                n177 = Or(x=w314, y=w313) -> (x .or. y?=w312:bool)
                n178 = case shown="True" w312 {
                  frame False {
                  }
                  frame True {
                    n179 = while {
                      stop <- w316 stop-if-true
                      n180 = local read "STOP"() -> (w317:bool)
                      n181 = local read "Frame Is Done"() -> (w318:bool)
                      n182 = Or(x=w318, y=w317) -> (x .or. y?=w316:bool)
                      n183 = Wait (ms)(milliseconds to wait=u32 1) -> ()  [unwired: 1 out]
                    }
                  }
                }
              }
              frame #1 {
                n184 = case shown="True" w320 {
                  tunnel: w321 -> [_ w324]
                  frame False {
                  }
                  frame True {
                    n185 = stacked-sequence {
                      tunnel: w324 -> [w327 w330]
                      frame #0 {
                        n186 = xnode "Read/Write Control"("FPGA VI Reference In"=w327, "RS"=TRUE) -> ()  [unwired: 1 in, 2 out]
                        n187 = Wait (ms)(milliseconds to wait=u32 1) -> ()  [unwired: 1 out]
                      }
                      frame #1 {
                        n188 = xnode "Read/Write Control"("FPGA VI Reference In"=w330, "RS"=FALSE) -> ()  [unwired: 1 in, 2 out]
                        n189 = Wait (ms)(milliseconds to wait=u32 1) -> ()  [unwired: 1 out]
                      }
                    }
                  }
                }
                n190 = case shown="True" w319 {
                  frame False {
                  }
                  frame True {
                    n191 = local read "Счетчик ОС"() -> (w323:u32)
                    n192 = Increment(x=w323) -> (x+1=→"Счетчик ОС":u32)
                  }
                }
              }
            }
          }
          frame #1 {
            n193 = local write "PreCapture"(TRUE ("PreCapture")) -> ()
            n194 = local write "Start"(FALSE ("Start")) -> ()
            n195 = Wait (ms)(milliseconds to wait=u32 5) -> ()  [unwired: 1 out]
          }
          frame #2 {
            w334 = FALSE ("RS")
            n196 = while {
              stop <- w337 stop-if-true
              n197 = local read "PreCaptureIsDone"() -> (w336:bool)
              n198 = local read "STOP"() -> (w335:bool)
              n199 = Wait (ms)(milliseconds to wait=u32 1) -> ()  [unwired: 1 out]
              n200 = Or(x=w336, y=w335) -> (x .or. y?=w337:bool)
            }
            n201 = local write "RS"(w334) -> ()
            n202 = local write "ОС"(w334) -> ()
          }
        }
      }
    }
    n203 = local read "STOP"() -> (w294:bool)
  }
  n204 = while {
    tunnel: w9 -> [w339]
    tunnel: w3 -> [_]
    stop <- w340 stop-if-true
    # "Предпрошивка перед принятием кадра. Необходимо после включения питания и после цифрового сброса"
    n205 = Wait (ms)(milliseconds to wait=u32 1) -> ()  [unwired: 1 out]
    n206 = case shown="True" "PreCapture" {
      tunnel: [w343 w345] -> w340
      tunnel: w339 -> [_ w344]
      frame False {
        n207 = local read "STOP"() -> (w343:bool)
      }
      frame True {
        n208 = stacked-sequence {
          tunnel: [_ _ w393] -> w345
          tunnel: w344 -> [w349 w373 _]
          frame #0 {
            n209 = flat-sequence {
              tunnel: w349 -> [w353]
              tunnel: [w350] -> w346
              tunnel: [w358] -> w347
              tunnel: w346 -> [w358]
              tunnel: [w361] -> w348
              tunnel: w347 -> [w361]
              tunnel: w348 -> [w367]
              frame #0 {
                n210 = local write "PreCapture"(FALSE ("FramePreCapture")) -> ()
                n211 = xnode "Read/Write Control"("FPGA VI Reference In"=w353, "CSTop"=TRUE, "CSBot"=FALSE) -> ("FPGA VI Reference Out"=w350:refnum<k20>)  [unwired: 1 in, 1 out]
                n212 = local write "Этап прошивки"(T2."CSTop" ("Этап прошивки")) -> ()
                n213 = Wait (ms)(milliseconds to wait=u32 3) -> ()  [unwired: 1 out]
                "PreCaptureIsDone" <- FALSE ("FirmwareIsDone")
              }
              frame #1 {
                n214 = local write "Firmware"(TRUE ("Firmware")) -> ()
                n215 = Wait (ms)(milliseconds to wait=u32 3) -> ()  [unwired: 1 out]
              }
              frame #2 {
                n216 = while {
                  stop <- w364 stop-if-true
                  n217 = local read "FirmwareIsDone"() -> (w363:bool)
                  n218 = local read "STOP"() -> (w362:bool)
                  n219 = Wait (ms)(milliseconds to wait=u32 1) -> ()  [unwired: 1 out]
                  n220 = Or(x=w363, y=w362) -> (x .or. y?=w364:bool)
                }
              }
              frame #3 {
                n221 = xnode "Read/Write Control"("FPGA VI Reference In"=w367, "CSTop"=FALSE, "CSBot"=FALSE) -> ()  [unwired: 1 in, 2 out]
                n222 = Wait (ms)(milliseconds to wait=u32 10) -> ()  [unwired: 1 out]
              }
            }
          }
          frame #1 {
            n223 = flat-sequence {
              tunnel: w373 -> [w377]
              tunnel: [w374] -> w372
              tunnel: w372 -> [w380]
              tunnel: [w380] -> w370
              tunnel: [w383] -> w371
              tunnel: w370 -> [w383]
              tunnel: w371 -> [w388]
              frame #0 {
                n224 = xnode "Read/Write Control"("FPGA VI Reference In"=w377, "CSTop"=FALSE, "CSBot"=TRUE) -> ("FPGA VI Reference Out"=w374:refnum<k20>)  [unwired: 1 in, 1 out]
                n225 = local write "Этап прошивки"(T2."CSBot" ("Этап прошивки")) -> ()
                n226 = Wait (ms)(milliseconds to wait=u32 5) -> ()  [unwired: 1 out]
              }
              frame #1 {
                n227 = local write "Firmware"(TRUE ("Firmware")) -> ()
                n228 = Wait (ms)(milliseconds to wait=u32 5) -> ()  [unwired: 1 out]
              }
              frame #2 {
                n229 = while {
                  stop <- w386 stop-if-true
                  n230 = local read "FirmwareIsDone"() -> (w385:bool)
                  n231 = local read "STOP"() -> (w384:bool)
                  n232 = Wait (ms)(milliseconds to wait=u32 1) -> ()  [unwired: 1 out]
                  n233 = Or(x=w385, y=w384) -> (x .or. y?=w386:bool)
                }
              }
              frame #3 {
                n234 = local write "PreCaptureIsDone"(TRUE ("FramePreCaptureIsDone")) -> ()
                n235 = xnode "Read/Write Control"("FPGA VI Reference In"=w388, "CSTop"=FALSE, "CSBot"=FALSE) -> ()  [unwired: 1 in, 2 out]
                n236 = Wait (ms)(milliseconds to wait=u32 1) -> ()  [unwired: 1 out]
              }
            }
          }
          frame #2 {
            n237 = local read "STOP"() -> (w393:bool)
          }
        }
      }
    }
  }
  n238 = while {
    tunnel: [w399] -> _
    tunnel: w20 -> [w397]
    tunnel: w19 -> [w396]
    tunnel: w3 -> [_]
    tunnel: [w395] -> w12
    tunnel: [w394] -> w11
    stop <- w399 stop-if-true
    # "Инициализация источников"
    n239 = Wait (ms)(milliseconds to wait=u32 1) -> ()  [unwired: 1 out]
    n240 = flat-sequence {
      tunnel: [w445] -> w399
      tunnel: w397 -> [w408]
      tunnel: w396 -> [w407]
      tunnel: [w406] -> w395
      tunnel: [w405] -> w394
      frame #0 {
        w412 = T9 0 items=["Current", "Voltage"] ("measurement type")
        n241 = local read "Power OFF"() -> (w404:bool)
        n242 = call <instrlib>:"niDCPower Configure Current Limit.vi"("current limit"="VDDD_curlim, A", "channel name"="0", "instrument handle"=w408) -> ("instrument handle out"=w459:refnum<k15>)  [unwired: 7 in, 1 out]
        n243 = call <instrlib>:"niDCPower Configure Current Limit.vi"("current limit"="VDDA_curlim, A", "channel name"="1", "instrument handle"=w408) -> ("instrument handle out"=w456:refnum<k15>)  [unwired: 7 in, 1 out]
        n244 = call <instrlib>:"niDCPower Configure Current Limit.vi"("current limit"="LED IR_curlim, A", "channel name"="2", "instrument handle"=w408) -> ("instrument handle out"=w418:refnum<k15>)  [unwired: 7 in, 1 out]
        n245 = call <instrlib>:"niDCPower Configure Current Limit.vi"("current limit"="+6, A", "channel name"="0", "instrument handle"=w407) -> ("instrument handle out"=w439:refnum<k15>)  [unwired: 7 in, 1 out]
        n246 = call <instrlib>:"niDCPower Configure Current Limit.vi"("current limit"="+0.5_curlim, A", "channel name"="1", "instrument handle"=w407) -> ("instrument handle out"=w428:refnum<k15>)  [unwired: 7 in, 1 out]
        n247 = call <instrlib>:"niDCPower Configure Voltage Level.vi"("voltage level"="VDDD, V", "channel name"="0", "instrument handle"=w459) -> ("instrument handle out"=w464:refnum<k15>)  [unwired: 7 in, 1 out]
        n248 = call <instrlib>:"niDCPower Configure Voltage Level.vi"("voltage level"="VDDA, V", "channel name"="1", "instrument handle"=w456) -> ("error out"=w462:errorcluster, "instrument handle out"=w463:refnum<k15>)  [unwired: 7 in]
        n249 = call <instrlib>:"niDCPower Configure Voltage Level.vi"("voltage level"="LED IR, V", "channel name"="2", "instrument handle"=w418) -> ("instrument handle out"=w421:refnum<k15>)  [unwired: 7 in, 1 out]
        n250 = call <instrlib>:"niDCPower Configure Voltage Level.vi"("voltage level"="+6, V", "channel name"="0", "instrument handle"=w439) -> ("instrument handle out"=w436:refnum<k15>)  [unwired: 7 in, 1 out]
        n251 = call <instrlib>:"niDCPower Configure Voltage Level.vi"("voltage level"="+0.5, V", "channel name"="1", "instrument handle"=w428) -> ("error out"=w431:errorcluster, "instrument handle out"=w432:refnum<k15>)  [unwired: 7 in]
        n252 = Select(t=FALSE, s=w404, f="LED IR ON") -> (s? t:f=w400:bool)
        n253 = call <instrlib>:"niDCPower Configure Output Enabled.vi"("output enabled"="VDDD ON", "channel name"="0", "instrument handle"=w464) -> ("instrument handle out"=w465:refnum<k15>)  [unwired: 7 in, 1 out]
        n254 = call <instrlib>:"niDCPower Configure Output Enabled.vi"("error in (no error)"=w462, "output enabled"="VDDA ON", "channel name"="1", "instrument handle"=w463) -> ("error out"=w467:errorcluster, "instrument handle out"=w466:refnum<k15>)  [unwired: 6 in]
        n255 = call <instrlib>:"niDCPower Configure Output Enabled.vi"("output enabled"=w400, "channel name"="2", "instrument handle"=w421) -> ("instrument handle out"=w422:refnum<k15>)  [unwired: 7 in, 1 out]
        n256 = call <instrlib>:"niDCPower Configure Output Enabled.vi"("output enabled"="+6 ON", "channel name"="0", "instrument handle"=w436) -> ("instrument handle out"=w435:refnum<k15>)  [unwired: 7 in, 1 out]
        n257 = call <instrlib>:"niDCPower Configure Output Enabled.vi"("error in (no error)"=w431, "output enabled"="+0.5 ON", "channel name"="1", "instrument handle"=w432) -> ("error out"=w434:errorcluster, "instrument handle out"=w433:refnum<k15>)  [unwired: 6 in]
        n258 = call <instrlib>:"niDCPower Measure.vi"("measurement type"=w412, "channel name"="0", "instrument handle"=w465) -> ("measurement"=→"VDDD_cur, A" →"VDDD_char":dbl, "instrument handle out"=w406:refnum<k15>)  [unwired: 6 in, 1 out]
        n259 = call <instrlib>:"niDCPower Measure.vi"("error in (no error)"=w467, "measurement type"=w412, "channel name"="1", "instrument handle"=w466) -> ("measurement"=→"VDDA_cur, A" →"VDDA_char":dbl)  [unwired: 5 in, 2 out]
        n260 = call <instrlib>:"niDCPower Measure.vi"("measurement type"=w412, "channel name"="2", "instrument handle"=w422) -> ("measurement"=→"LED IR_cur, A" →"LED IR_char":dbl)  [unwired: 6 in, 2 out]
        n261 = call <instrlib>:"niDCPower Measure.vi"("measurement type"=w412, "channel name"="0", "instrument handle"=w435) -> ("measurement"=→"+6_cur, A" →"+6_char":dbl, "instrument handle out"=w405:refnum<k15>)  [unwired: 6 in, 1 out]
        n262 = call <instrlib>:"niDCPower Measure.vi"("error in (no error)"=w434, "measurement type"=w412, "channel name"="1", "instrument handle"=w433) -> ("measurement"=→"+0.5_cur, A" →"+0,5_char":dbl)  [unwired: 5 in, 2 out]
        n263 = local read "Power OFF"() -> (w445:bool)
      }
    }
  }
  n264 = while {
    shift-right: ["Save"] -> _
    shift-left: FALSE ("Сохранить") -> [w471]
    tunnel: [w468] -> _
    tunnel: w3 -> [_]
    stop <- w468 stop-if-true
    n265 = Wait (ms)(milliseconds to wait=u32 1) -> ()  [unwired: 1 out]
    n266 = Greater?(x="Save", y=w471) -> (0:w472:bool)
    n267 = case shown="True" w472 {
      frame False {
      }
      frame True {
        n268 = local read "Test Model Log Path"() -> (w473:path)
        n269 = Build Path(base path=w473, name or relative path="Frames") -> (appended path=w495:path)
        n270 = call <vilib>:"Check if File or Folder Exists.vi"("path"=w495) -> ("file or folder exists?"=w494:bool, "dup path"=w493:path)  [unwired: 8 in, 1 out]
        n271 = case shown="False" w494 {
          tunnel: w493 -> [w500 w501]
          tunnel: [w499 w501] -> w483
          frame False {
            n272 = Create Folder(path (use dialog)=w500) -> (created path=w499:path)  [unwired: 2 in, 2 out]
          }
          frame True {
          }
        }
        n273 = Select(t="Светло", s="Темный(F)\nСветлый(T)", f="Темно") -> (s? t:f=w479:string)
        n274 = Build Path(base path=w483, name or relative path=w479) -> (appended path=w484:path)
        n275 = Get Date/Time In Seconds() -> (seconds since 1Jan1904=w492:timestamp)
        n276 = call <vilib>:"Check if File or Folder Exists.vi"("path"=w484) -> ("file or folder exists?"=w485:bool, "dup path"=w486:path)  [unwired: 8 in, 1 out]
        n277 = Format Date/Time String(time format string (%c)="%d %H.%M.%S", seconds (now)=w492) -> (date/time string=w491:string)  [unwired: 1 in]
        n278 = case shown="False" w485 {
          tunnel: w486 -> [w497 w498]
          tunnel: [w496 w498] -> w478
          frame False {
            n279 = Create Folder(path (use dialog)=w497) -> (created path=w496:path)  [unwired: 2 in, 2 out]
          }
          frame True {
          }
        }
        n280 = Concatenate Strings(w491, "_" ("string"), "Примечание", ".tiff" ("string")) -> (w477:string)
        n281 = local read "Image"() -> (w475:T3)
        n282 = Build Path(base path=w478, name or relative path=w477) -> (appended path=w476:path)
        n283 = call-poly "IMAQ Write File 2"("File Path"=w476, "Image"=w475) -> ()  [unwired: 8 in, 2 out]
      }
    }
    n284 = local read "STOP"() -> (w468:bool)
  }
  n285 = while {
    tunnel: w9 -> [w505]
    tunnel: w3 -> [_]
    stop <- w503 stop-if-true
    # "Драйвер прошивки матрицы"
    n286 = Wait (ms)(milliseconds to wait=u32 1) -> ()  [unwired: 1 out]
    n287 = case shown="True" "Firmware" {
      tunnel: "Этап прошивки" -> [_ w510]
      tunnel: w505 -> [_ w509]
      tunnel: [w507 w508] -> w503
      frame False {
        n288 = local read "STOP"() -> (w507:bool)
      }
      frame True {
        n289 = stacked-sequence {
          tunnel: w510 -> [w516 _ _]
          tunnel: w509 -> [w515 w549 _]
          tunnel: [_ _ w577] -> w508
          frame #0 {
            n290 = flat-sequence {
              tunnel: w516 -> [w522]
              tunnel: w515 -> [w521]
              tunnel: [w519] -> w514
              tunnel: w514 -> [w526]
              tunnel: [w525] -> w512
              tunnel: [w527] -> w513
              tunnel: w512 -> [w528]
              tunnel: w513 -> [w538]
              tunnel: [w537] -> w511
              tunnel: w511 -> [w539]
              frame #0 {
                n291 = xnode "Read/Write Control"("FPGA VI Reference In"=w521, "Этап прошивки"=w522) -> ("FPGA VI Reference Out"=w519:refnum<k20>)  [unwired: 1 in, 1 out]
                n292 = local write "Firmware"(FALSE ("Firmware")) -> ()
                n293 = Wait (ms)(milliseconds to wait=u32 1) -> ()  [unwired: 1 out]
                "FirmwareIsDone" <- FALSE ("FirmwareIsDone")
              }
              frame #1 {
                n294 = xnode "Read/Write Control"("FPGA VI Reference In"=w526, "SetReg"=TRUE) -> ("FPGA VI Reference Out"=w525:refnum<k20>)  [unwired: 1 in, 1 out]
                n295 = Wait (ms)(milliseconds to wait=u32 1) -> ()  [unwired: 1 out]
              }
              frame #2 {
                n296 = while {
                  tunnel: w528 -> [w533]
                  tunnel: [w532] -> w527
                  stop <- w531 stop-if-true
                  n297 = xnode "Read/Write Control"("FPGA VI Reference In"=w533) -> ("FPGA VI Reference Out"=w532:refnum<k20>, "SetRegIsDone"=w530:bool)  [unwired: 1 in, 1 out]
                  n298 = local read "STOP"() -> (w529:bool)
                  n299 = Wait (ms)(milliseconds to wait=u32 1) -> ()  [unwired: 1 out]
                  n300 = Or(x=w530, y=w529) -> (x .or. y?=w531:bool)
                }
              }
              frame #3 {
                n301 = xnode "Read/Write Control"("FPGA VI Reference In"=w538, "ResetSetReg"=TRUE ("ReseSetReg")) -> ("FPGA VI Reference Out"=w537:refnum<k20>)  [unwired: 1 in, 1 out]
                n302 = Wait (ms)(milliseconds to wait=u32 1) -> ()  [unwired: 1 out]
              }
              frame #4 {
                n303 = while {
                  tunnel: w539 -> [w545]
                  stop <- w540 stop-if-true
                  n304 = xnode "Read/Write Control"("FPGA VI Reference In"=w545) -> ("FPGA VI Reference Out"=w544:refnum<k20>, "SetRegIsDone"=w542:bool)  [unwired: 1 in, 1 out]
                  n305 = Wait (ms)(milliseconds to wait=u32 1) -> ()  [unwired: 1 out]
                  n306 = local read "STOP"() -> (w543:bool)
                  n307 = Not(x=w542) -> (.not. x?=w541:bool)
                  n308 = xnode "Read/Write Control"("FPGA VI Reference In"=w544, "ResetSetReg"=w542) -> ()  [unwired: 1 in, 2 out]
                  n309 = Or(x=w541, y=w543) -> (x .or. y?=w540:bool)
                }
              }
            }
          }
          frame #1 {
            n310 = flat-sequence {
              tunnel: [w552] -> w550
              tunnel: w549 -> [w553]
              tunnel: w550 -> [w556]
              tunnel: [w555] -> w547
              tunnel: [w565] -> w548
              tunnel: w547 -> [w566]
              tunnel: w548 -> [w567]
              frame #0 {
                n311 = xnode "Read/Write Control"("FPGA VI Reference In"=w553, "SendData"=TRUE) -> ("FPGA VI Reference Out"=w552:refnum<k20>)  [unwired: 1 in, 1 out]
                n312 = Wait (ms)(milliseconds to wait=u32 1) -> ()  [unwired: 1 out]
              }
              frame #1 {
                n313 = while {
                  tunnel: w556 -> [w558]
                  tunnel: [w557] -> w555
                  stop <- w561 stop-if-true
                  n314 = local read "STOP"() -> (w560:bool)
                  n315 = xnode "Read/Write Control"("FPGA VI Reference In"=w558) -> ("FPGA VI Reference Out"=w557:refnum<k20>, "SendDataIsDone"=w559:bool)  [unwired: 1 in, 1 out]
                  n316 = Wait (ms)(milliseconds to wait=u32 1) -> ()  [unwired: 1 out]
                  n317 = Or(x=w559, y=w560) -> (x .or. y?=w561:bool)
                }
              }
              frame #2 {
                n318 = xnode "Read/Write Control"("FPGA VI Reference In"=w566, "ResetSendData"=TRUE ("ReseSendData")) -> ("FPGA VI Reference Out"=w565:refnum<k20>)  [unwired: 1 in, 1 out]
                n319 = Wait (ms)(milliseconds to wait=u32 1) -> ()  [unwired: 1 out]
              }
              frame #3 {
                n320 = while {
                  tunnel: w567 -> [w573]
                  stop <- w570 stop-if-true
                  n321 = xnode "Read/Write Control"("FPGA VI Reference In"=w573) -> ("FPGA VI Reference Out"=w572:refnum<k20>, "SendDataIsDone"=w568:bool)  [unwired: 1 in, 1 out]
                  n322 = Wait (ms)(milliseconds to wait="Задержка прошивки") -> ()  [unwired: 1 out]
                  n323 = local read "STOP"() -> (w569:bool)
                  n324 = Not(x=w568) -> (.not. x?=w571:bool)
                  n325 = Or(x=w571, y=w569) -> (x .or. y?=w570:bool)
                  n326 = xnode "Read/Write Control"("FPGA VI Reference In"=w572, "ResetSendData"=w568) -> ()  [unwired: 1 in, 2 out]
                }
              }
              frame #4 {
                n327 = local write "FirmwareIsDone"(TRUE ("FirmwareIsDone")) -> ()
                n328 = Wait (ms)(milliseconds to wait=u32 1) -> ()  [unwired: 1 out]
              }
            }
          }
          frame #2 {
            n329 = local read "STOP"() -> (w577:bool)
          }
        }
      }
    }
  }
  n330 = while {
    tunnel: w9 -> [w580]
    shift-right: ["Прошить АЦП"] -> _
    shift-left: FALSE ("Прошить АЦП") -> [w586]
    tunnel: w3 -> [_]
    stop <- w587 stop-if-true
    # "Драйвер прошивки АЦП"
    n331 = local read "STOP"() -> (w583:bool)
    n332 = Greater?(x="Прошить АЦП", y=w586) -> (0:w584:bool)
    n333 = Wait (ms)(milliseconds to wait=u32 1) -> ()  [unwired: 1 out]
    n334 = Not(x=w583) -> (.not. x?=w582:bool)
    n335 = And(x=w582, y=w584) -> (x .and. y?=w578:bool)
    n336 = case shown="True" w578 {
      tunnel: "ADC Register Map" -> [_ w589]
      tunnel: w580 -> [_ w588]
      frame False {
      }
      frame True {
        n337 = stacked-sequence {
          tunnel: w589 -> [_ w592 _]
          tunnel: w588 -> [_ w591 _]
          frame #0 {
            "АЦП прошит!" <- FALSE ("АЦП прошит!")
          }
          frame #1 {
            n338 = case shown="\"MUX\"" w592 {
              selector: w592 -> [w596 w654 w686 w711 w736 w760 w790 w819]
              tunnel: w591 -> [w595 w653 w685 w710 w735 w761 w789 w818]
              frame "Configuration", Default {
                w599 = FALSE
                # "SHA Mode"
                # "8"
                # "0"
                # "Configuration"
                n339 = xnode "Read/Write Control"("FPGA VI Reference In"=w595, "Enum"=w596) -> ("FPGA VI Reference Out"=w610:refnum<k20>)  [unwired: 1 in, 1 out]
                n340 = case shown="\"4V\"" "2/4 V" {
                  tunnel: [FALSE TRUE] -> w604
                  frame "2V", Default {
                  }
                  frame "4V" {
                  }
                }
                n341 = case shown="\"1CH\"" "3CH/1CH" {
                  tunnel: [TRUE FALSE] -> w603
                  frame "3CH", Default {
                  }
                  frame "1CH" {
                  }
                }
                n342 = xnode "Read/Write Control"("FPGA VI Reference In"=w618, "Read(T)/Write(F)"=TRUE) -> ("FPGA VI Reference Out"=w612:refnum<k20>, "error out"=w613:errorcluster)  [unwired: 1 in]
                n343 = xnode "Read/Write Control"("FPGA VI Reference In"=w610, "Read(T)/Write(F)"=FALSE) -> ("FPGA VI Reference Out"=w611:refnum<k20>)  [unwired: 1 in, 1 out]
                n344 = Build Array(w599, w599, w599, TRUE ("element"), FALSE, w603, TRUE ("element"), w604, FALSE) -> (w602:bool[])
                n345 = flat-sequence {
                  tunnel: w612 -> [w631]
                  tunnel: w613 -> [w630]
                  tunnel: [w629] -> w614
                  tunnel: [w628] -> w615
                  frame #0 {
                    n346 = xnode "Read/Write Control"("FPGA VI Reference In"=w631, "error in"=w630, "Конфигурация"=TRUE) -> ("FPGA VI Reference Out"=w629:refnum<k20>, "error out"=w628:errorcluster)
                    n347 = Wait (ms)(milliseconds to wait=u32 10) -> ()  [unwired: 1 out]
                  }
                }
                n348 = Reverse 1D Array(array=w602) -> (reversed array=w607:bool[])
                n349 = xnode "Read/Write Control"("FPGA VI Reference In"=w611, "Write Data"=w607) -> ("FPGA VI Reference Out"=w608:refnum<k20>)  [unwired: 1 in, 1 out]
                n350 = flat-sequence {
                  tunnel: w614 -> [w625]
                  tunnel: w615 -> [w624]
                  tunnel: [w622] -> w616
                  tunnel: [w621] -> w617
                  frame #0 {
                    n351 = xnode "Read/Write Control"("FPGA VI Reference In"=w625, "error in"=w624, "Конфигурация"=FALSE) -> ("FPGA VI Reference Out"=w622:refnum<k20>, "error out"=w621:errorcluster)
                    n352 = Wait (ms)(milliseconds to wait=u32 10) -> ()  [unwired: 1 out]
                  }
                }
                n353 = flat-sequence {
                  tunnel: w608 -> [w639]
                  tunnel: [w637] -> w609
                  frame #0 {
                    n354 = xnode "Read/Write Control"("FPGA VI Reference In"=w639, "Конфигурация"=TRUE) -> ("FPGA VI Reference Out"=w637:refnum<k20>)  [unwired: 1 in, 1 out]
                    n355 = Wait (ms)(milliseconds to wait=u32 10) -> ()  [unwired: 1 out]
                  }
                }
                n356 = xnode "Read/Write Control"("FPGA VI Reference In"=w616, "error in"=w617) -> ("READ"=→"Configuration":bool[])  [unwired: 2 out]
                n357 = flat-sequence {
                  tunnel: w609 -> [w635]
                  tunnel: [w633] -> w618
                  frame #0 {
                    n358 = xnode "Read/Write Control"("FPGA VI Reference In"=w635, "Конфигурация"=FALSE) -> ("FPGA VI Reference Out"=w633:refnum<k20>)  [unwired: 1 in, 1 out]
                    n359 = Wait (ms)(milliseconds to wait=u32 10) -> ()  [unwired: 1 out]
                  }
                }
              }
              frame "MUX" {
                # "MUX"
                n360 = xnode "Read/Write Control"("FPGA VI Reference In"=w644, "Read(T)/Write(F)"=TRUE) -> ("FPGA VI Reference Out"=w646:refnum<k20>, "error out"=w647:errorcluster)  [unwired: 1 in]
                n361 = xnode "Read/Write Control"("FPGA VI Reference In"=w653, "Enum"=w654) -> ("FPGA VI Reference Out"=w659:refnum<k20>)  [unwired: 1 in, 1 out]
                n362 = case shown="\"RED\", Default" "Какой канал?" {
                  tunnel: [bool[] [FALSE, TRUE, FALSE, TRUE, FALSE, FALSE, FALSE, FALSE, FALSE] ("MUX_register") bool[] [FALSE, TRUE, TRUE, FALSE, FALSE, FALSE, FALSE, FALSE, FALSE] ("MUX_register") bool[] [FALSE, TRUE, FALSE, FALSE, TRUE, FALSE, FALSE, FALSE, FALSE] ("MUX_register")] -> w661
                  frame "GREEN" {
                  }
                  frame "RED", Default {
                  }
                  frame "BLUE" {
                  }
                }
                n363 = xnode "Read/Write Control"("FPGA VI Reference In"=w659, "Read(T)/Write(F)"=FALSE) -> ("FPGA VI Reference Out"=w658:refnum<k20>)  [unwired: 1 in, 1 out]
                n364 = flat-sequence {
                  tunnel: w646 -> [w673]
                  tunnel: w647 -> [w672]
                  tunnel: [w671] -> w648
                  tunnel: [w670] -> w649
                  frame #0 {
                    n365 = xnode "Read/Write Control"("FPGA VI Reference In"=w673, "error in"=w672, "Конфигурация"=TRUE) -> ("FPGA VI Reference Out"=w671:refnum<k20>, "error out"=w670:errorcluster)
                    n366 = Wait (ms)(milliseconds to wait=u32 10) -> ()  [unwired: 1 out]
                  }
                }
                n367 = xnode "Read/Write Control"("FPGA VI Reference In"=w658, "Write Data"=w661) -> ("FPGA VI Reference Out"=w657:refnum<k20>)  [unwired: 1 in, 1 out]
                n368 = flat-sequence {
                  tunnel: w648 -> [w667]
                  tunnel: w649 -> [w666]
                  tunnel: [w664] -> w650
                  tunnel: [w663] -> w651
                  frame #0 {
                    n369 = xnode "Read/Write Control"("FPGA VI Reference In"=w667, "error in"=w666, "Конфигурация"=FALSE) -> ("FPGA VI Reference Out"=w664:refnum<k20>, "error out"=w663:errorcluster)
                    n370 = Wait (ms)(milliseconds to wait=u32 10) -> ()  [unwired: 1 out]
                  }
                }
                n371 = flat-sequence {
                  tunnel: [w683] -> w656
                  tunnel: w657 -> [w682]
                  frame #0 {
                    n372 = xnode "Read/Write Control"("FPGA VI Reference In"=w682, "Конфигурация"=TRUE) -> ("FPGA VI Reference Out"=w683:refnum<k20>)  [unwired: 1 in, 1 out]
                    n373 = Wait (ms)(milliseconds to wait=u32 10) -> ()  [unwired: 1 out]
                  }
                }
                n374 = flat-sequence {
                  tunnel: w656 -> [w680]
                  tunnel: [w678] -> w644
                  frame #0 {
                    n375 = xnode "Read/Write Control"("FPGA VI Reference In"=w680, "Конфигурация"=FALSE) -> ("FPGA VI Reference Out"=w678:refnum<k20>)  [unwired: 1 in, 1 out]
                    n376 = Wait (ms)(milliseconds to wait=u32 10) -> ()  [unwired: 1 out]
                  }
                }
                n377 = xnode "Read/Write Control"("FPGA VI Reference In"=w650, "error in"=w651) -> ("READ"=→"MUX":bool[])  [unwired: 2 out]
              }
              frame "RED PGA" {
                w688 = FALSE
                # "RED PGA"
                n378 = Decrement(x="Усиление (до 6)_RED") -> (x-1=w700:u8)
                n379 = Multiply(x=w700, y=378) -> (x*y=w699:i32)
                n380 = Multiply(x="Усиление (до 6)_RED", y=5) -> (x*y=w697:i32)
                n381 = xnode "Read/Write Control"("FPGA VI Reference In"=w685, "Enum"=w686) -> ("FPGA VI Reference Out"=w693:refnum<k20>)  [unwired: 1 in, 1 out]
                n382 = Divide(x=w699, y=w697) -> (x/y=w696:dbl)
                n383 = Number To Boolean Array(number=w696) -> (Boolean array=w701:bool[])
                n384 = xnode "Read/Write Control"("FPGA VI Reference In"=w693, "Read(T)/Write(F)"=FALSE) -> ("FPGA VI Reference Out"=w694:refnum<k20>)  [unwired: 1 in, 1 out]
                n385 = Build Array (concatenate)(w688, w688, w688, w701) -> (w695:bool[])
                n386 = xnode "Read/Write Control"("FPGA VI Reference In"=w694, "Write Data"=w695) -> ("FPGA VI Reference Out"=w692:refnum<k20>)  [unwired: 1 in, 1 out]
                n387 = flat-sequence {
                  tunnel: [w708] -> w691
                  tunnel: w692 -> [w707]
                  frame #0 {
                    n388 = xnode "Read/Write Control"("FPGA VI Reference In"=w707, "Конфигурация"=TRUE) -> ("FPGA VI Reference Out"=w708:refnum<k20>)  [unwired: 1 in, 1 out]
                    n389 = Wait (ms)(milliseconds to wait=u32 10) -> ()  [unwired: 1 out]
                  }
                }
                n390 = flat-sequence {
                  tunnel: w691 -> [w705]
                  tunnel: [w703] -> _
                  frame #0 {
                    n391 = xnode "Read/Write Control"("FPGA VI Reference In"=w705, "Конфигурация"=FALSE) -> ("FPGA VI Reference Out"=w703:refnum<k20>)  [unwired: 1 in, 1 out]
                    n392 = Wait (ms)(milliseconds to wait=u32 10) -> ()  [unwired: 1 out]
                  }
                }
              }
              frame "GREEN PGA" {
                w713 = FALSE
                # "GREEN PGA"
                n393 = Decrement(x="Усиление (до 6)_GREEN") -> (x-1=w725:u8)
                n394 = Multiply(x=w725, y=378) -> (x*y=w724:i32)
                n395 = Multiply(x="Усиление (до 6)_GREEN", y=5) -> (x*y=w722:i32)
                n396 = xnode "Read/Write Control"("FPGA VI Reference In"=w710, "Enum"=w711) -> ("FPGA VI Reference Out"=w718:refnum<k20>)  [unwired: 1 in, 1 out]
                n397 = Divide(x=w724, y=w722) -> (x/y=w721:dbl)
                n398 = Number To Boolean Array(number=w721) -> (Boolean array=w726:bool[])
                n399 = xnode "Read/Write Control"("FPGA VI Reference In"=w718, "Read(T)/Write(F)"=FALSE) -> ("FPGA VI Reference Out"=w719:refnum<k20>)  [unwired: 1 in, 1 out]
                n400 = Build Array (concatenate)(w713, w713, w713, w726) -> (w720:bool[])
                n401 = xnode "Read/Write Control"("FPGA VI Reference In"=w719, "Write Data"=w720) -> ("FPGA VI Reference Out"=w717:refnum<k20>)  [unwired: 1 in, 1 out]
                n402 = flat-sequence {
                  tunnel: [w733] -> w716
                  tunnel: w717 -> [w732]
                  frame #0 {
                    n403 = xnode "Read/Write Control"("FPGA VI Reference In"=w732, "Конфигурация"=TRUE) -> ("FPGA VI Reference Out"=w733:refnum<k20>)  [unwired: 1 in, 1 out]
                    n404 = Wait (ms)(milliseconds to wait=u32 10) -> ()  [unwired: 1 out]
                  }
                }
                n405 = flat-sequence {
                  tunnel: w716 -> [w730]
                  tunnel: [w728] -> _
                  frame #0 {
                    n406 = xnode "Read/Write Control"("FPGA VI Reference In"=w730, "Конфигурация"=FALSE) -> ("FPGA VI Reference Out"=w728:refnum<k20>)  [unwired: 1 in, 1 out]
                    n407 = Wait (ms)(milliseconds to wait=u32 10) -> ()  [unwired: 1 out]
                  }
                }
              }
              frame "BLUE PGA" {
                w738 = FALSE
                # "BLUE PGA"
                n408 = Decrement(x="Усиление (до 6)_BLUE") -> (x-1=w750:u8)
                n409 = Multiply(x=w750, y=378) -> (x*y=w749:i32)
                n410 = Multiply(x="Усиление (до 6)_BLUE", y=5) -> (x*y=w747:i32)
                n411 = xnode "Read/Write Control"("FPGA VI Reference In"=w735, "Enum"=w736) -> ("FPGA VI Reference Out"=w743:refnum<k20>)  [unwired: 1 in, 1 out]
                n412 = Divide(x=w749, y=w747) -> (x/y=w746:dbl)
                n413 = Number To Boolean Array(number=w746) -> (Boolean array=w751:bool[])
                n414 = xnode "Read/Write Control"("FPGA VI Reference In"=w743, "Read(T)/Write(F)"=FALSE) -> ("FPGA VI Reference Out"=w744:refnum<k20>)  [unwired: 1 in, 1 out]
                n415 = Build Array (concatenate)(w738, w738, w738, w751) -> (w745:bool[])
                n416 = xnode "Read/Write Control"("FPGA VI Reference In"=w744, "Write Data"=w745) -> ("FPGA VI Reference Out"=w742:refnum<k20>)  [unwired: 1 in, 1 out]
                n417 = flat-sequence {
                  tunnel: [w758] -> w741
                  tunnel: w742 -> [w757]
                  frame #0 {
                    n418 = xnode "Read/Write Control"("FPGA VI Reference In"=w757, "Конфигурация"=TRUE) -> ("FPGA VI Reference Out"=w758:refnum<k20>)  [unwired: 1 in, 1 out]
                    n419 = Wait (ms)(milliseconds to wait=u32 10) -> ()  [unwired: 1 out]
                  }
                }
                n420 = flat-sequence {
                  tunnel: w741 -> [w755]
                  tunnel: [w753] -> _
                  frame #0 {
                    n421 = xnode "Read/Write Control"("FPGA VI Reference In"=w755, "Конфигурация"=FALSE) -> ("FPGA VI Reference Out"=w753:refnum<k20>)  [unwired: 1 in, 1 out]
                    n422 = Wait (ms)(milliseconds to wait=u32 10) -> ()  [unwired: 1 out]
                  }
                }
              }
              frame "RED OFF" {
                # "RED_OFFSET"
                n423 = case shown="\"-\", Default" "+/- RED" {
                  tunnel: [TRUE FALSE] -> w767
                  frame "-", Default {
                  }
                  frame "+" {
                  }
                }
                n424 = Quotient & Remainder(x="Смещение, до 300_RED", y=1.171875) -> (floor(x/y)=w772:dbl)  [unwired: 1 out]
                n425 = xnode "Read/Write Control"("FPGA VI Reference In"=w761, "Enum"=w760) -> ("FPGA VI Reference Out"=w776:refnum<k20>, "error out"=w775:errorcluster)  [unwired: 1 in]
                n426 = Subtract(x=w772, y=1.0) -> (x-y=w769:dbl)
                n427 = To Unsigned Byte Integer(number=w769) -> (unsigned 8bit integer=w768:u8)
                n428 = xnode "Read/Write Control"("FPGA VI Reference In"=w776, "error in"=w775, "Read(T)/Write(F)"=FALSE) -> ("FPGA VI Reference Out"=w774:refnum<k20>)  [unwired: 1 out]
                n429 = Number To Boolean Array(number=w768) -> (Boolean array=w766:bool[])
                n430 = Reverse 1D Array(array=w766) -> (reversed array=w765:bool[])
                n431 = Build Array (concatenate)(w767, w765) -> (w770:bool[])
                n432 = xnode "Read/Write Control"("FPGA VI Reference In"=w774, "Write Data"=w770) -> ("FPGA VI Reference Out"=w778:refnum<k20>)  [unwired: 1 in, 1 out]
                n433 = flat-sequence {
                  tunnel: w778 -> [w788]
                  tunnel: [w786] -> w777
                  frame #0 {
                    n434 = xnode "Read/Write Control"("FPGA VI Reference In"=w788, "Конфигурация"=TRUE) -> ("FPGA VI Reference Out"=w786:refnum<k20>)  [unwired: 1 in, 1 out]
                    n435 = Wait (ms)(milliseconds to wait=u32 10) -> ()  [unwired: 1 out]
                  }
                }
                n436 = flat-sequence {
                  tunnel: w777 -> [w784]
                  tunnel: [w782] -> _
                  frame #0 {
                    n437 = xnode "Read/Write Control"("FPGA VI Reference In"=w784, "Конфигурация"=FALSE) -> ("FPGA VI Reference Out"=w782:refnum<k20>)  [unwired: 1 in, 1 out]
                    n438 = Wait (ms)(milliseconds to wait=u32 10) -> ()  [unwired: 1 out]
                  }
                }
              }
              frame "GREEN OFF" {
                # "GREEN_OFFSET"
                n439 = case shown="\"-\", Default" "+/- GREEN" {
                  tunnel: [TRUE FALSE] -> w805
                  frame "-", Default {
                  }
                  frame "+" {
                  }
                }
                n440 = Quotient & Remainder(x="Смещение, до 300_GREEN", y=1.171875) -> (floor(x/y)=w800:dbl)  [unwired: 1 out]
                n441 = xnode "Read/Write Control"("FPGA VI Reference In"=w789, "Enum"=w790) -> ("FPGA VI Reference Out"=w796:refnum<k20>, "error out"=w797:errorcluster)  [unwired: 1 in]
                n442 = Subtract(x=w800, y=1.0) -> (x-y=w803:dbl)
                n443 = To Unsigned Byte Integer(number=w803) -> (unsigned 8bit integer=w804:u8)
                n444 = xnode "Read/Write Control"("FPGA VI Reference In"=w796, "error in"=w797, "Read(T)/Write(F)"=FALSE) -> ("FPGA VI Reference Out"=w798:refnum<k20>)  [unwired: 1 out]
                n445 = Number To Boolean Array(number=w804) -> (Boolean array=w806:bool[])
                n446 = Reverse 1D Array(array=w806) -> (reversed array=w807:bool[])
                n447 = Build Array (concatenate)(w805, w807) -> (w802:bool[])
                n448 = xnode "Read/Write Control"("FPGA VI Reference In"=w798, "Write Data"=w802) -> ("FPGA VI Reference Out"=w794:refnum<k20>)  [unwired: 1 in, 1 out]
                n449 = flat-sequence {
                  tunnel: w794 -> [w817]
                  tunnel: [w815] -> w795
                  frame #0 {
                    n450 = xnode "Read/Write Control"("FPGA VI Reference In"=w817, "Конфигурация"=TRUE) -> ("FPGA VI Reference Out"=w815:refnum<k20>)  [unwired: 1 in, 1 out]
                    n451 = Wait (ms)(milliseconds to wait=u32 10) -> ()  [unwired: 1 out]
                  }
                }
                n452 = flat-sequence {
                  tunnel: w795 -> [w813]
                  tunnel: [w811] -> _
                  frame #0 {
                    n453 = xnode "Read/Write Control"("FPGA VI Reference In"=w813, "Конфигурация"=FALSE) -> ("FPGA VI Reference Out"=w811:refnum<k20>)  [unwired: 1 in, 1 out]
                    n454 = Wait (ms)(milliseconds to wait=u32 10) -> ()  [unwired: 1 out]
                  }
                }
              }
              frame "BLUE OFF" {
                # "BLUE_OFFSET"
                n455 = case shown="\"-\", Default" "+/- BLUE" {
                  tunnel: [TRUE FALSE] -> w825
                  frame "-", Default {
                  }
                  frame "+" {
                  }
                }
                n456 = Quotient & Remainder(x="Смещение, до 300_BLUE", y=1.171875) -> (floor(x/y)=w830:dbl)  [unwired: 1 out]
                n457 = xnode "Read/Write Control"("FPGA VI Reference In"=w818, "Enum"=w819) -> ("FPGA VI Reference Out"=w834:refnum<k20>, "error out"=w833:errorcluster)  [unwired: 1 in]
                n458 = Subtract(x=w830, y=1.0) -> (x-y=w827:dbl)
                n459 = To Unsigned Byte Integer(number=w827) -> (unsigned 8bit integer=w826:u8)
                n460 = xnode "Read/Write Control"("FPGA VI Reference In"=w834, "error in"=w833, "Read(T)/Write(F)"=FALSE) -> ("FPGA VI Reference Out"=w832:refnum<k20>)  [unwired: 1 out]
                n461 = Number To Boolean Array(number=w826) -> (Boolean array=w824:bool[])
                n462 = Reverse 1D Array(array=w824) -> (reversed array=w823:bool[])
                n463 = Build Array (concatenate)(w825, w823) -> (w828:bool[])
                n464 = xnode "Read/Write Control"("FPGA VI Reference In"=w832, "Write Data"=w828) -> ("FPGA VI Reference Out"=w836:refnum<k20>)  [unwired: 1 in, 1 out]
                n465 = flat-sequence {
                  tunnel: w836 -> [w846]
                  tunnel: [w844] -> w835
                  frame #0 {
                    n466 = xnode "Read/Write Control"("FPGA VI Reference In"=w846, "Конфигурация"=TRUE) -> ("FPGA VI Reference Out"=w844:refnum<k20>)  [unwired: 1 in, 1 out]
                    n467 = Wait (ms)(milliseconds to wait=u32 10) -> ()  [unwired: 1 out]
                  }
                }
                n468 = flat-sequence {
                  tunnel: w835 -> [w842]
                  tunnel: [w840] -> _
                  frame #0 {
                    n469 = xnode "Read/Write Control"("FPGA VI Reference In"=w842, "Конфигурация"=FALSE) -> ("FPGA VI Reference Out"=w840:refnum<k20>)  [unwired: 1 in, 1 out]
                    n470 = Wait (ms)(milliseconds to wait=u32 10) -> ()  [unwired: 1 out]
                  }
                }
              }
            }
          }
          frame #2 {
            n471 = local write "АЦП прошит!"(TRUE ("АЦП прошит!")) -> ()
          }
        }
      }
    }
    n472 = local read "STOP"() -> (w587:bool)
  }
  n473 = while {
    tunnel: w9 -> [w850]
    tunnel: [w849] -> _
    tunnel: w3 -> [_]
    stop <- w848 stop-if-true
    # "Target"
    n474 = Wait (ms)(milliseconds to wait=u32 1) -> ()  [unwired: 1 out]
    n475 = xnode "Read/Write Control"("FPGA VI Reference In"=w850, "Автомат"="Автомат", "7..0(F)/0..7(T)"="7..0(F)/0..7(T)", "F(F)/R(T)_CmAD"="F(F)/R(T)_CmAD", "F(F)/R(T)_FIFO"="F(F)/R(T)_FIFO") -> ("FPGA VI Reference Out"=w849:refnum<k20>, "FIFOIsDone"=→"FIFOIsDone":bool)  [unwired: 1 in, 1 out]
    n476 = local read "STOP"() -> (w848:bool)
  }
  n477 = while {
    shift-right: ["Питание"] -> _
    shift-left: FALSE ("POWER") -> [w866]
    tunnel: w3 -> [_]
    stop <- w857 stop-if-true
    # "Включение / выключение образца и оснастки"
    n478 = Wait (ms)(milliseconds to wait=u32 1) -> ()  [unwired: 1 out]
    n479 = Less?(x="Питание", y=w866) -> (x < y?=w861:bool)
    n480 = Not(x="STOP") -> (.not. x?=w863:bool)
    n481 = Greater?(x="Питание", y=w866) -> (0:w862:bool)
    n482 = Or(x="STOP", y=w861) -> (x .or. y?=w860:bool)
    n483 = And(x=w863, y=w862) -> (x .and. y?=w864:bool)
    n484 = stacked-sequence {
      tunnel: w864 -> [w869]
      tunnel: w860 -> [w868]
      tunnel: [w867] -> w857
      tunnel: "STOP" -> [w867]
      frame #0 {
        n485 = case shown="True" w869 {
          frame False {
          }
          frame True {
            # "ON"
            n486 = flat-sequence {
              frame #0 {
                n487 = local write "VDDD ON"(TRUE ("VDDD ON")) -> ()
                n488 = Wait (ms)(milliseconds to wait=u32 100) -> ()  [unwired: 1 out]
              }
              frame #1 {
                w875 = TRUE ("VDDD ON")
                n489 = local write "VDDA ON"(w875) -> ()
                n490 = local write "+6 ON"(w875) -> ()
                n491 = local write "+0.5 ON"(w875) -> ()
                n492 = Wait (ms)(milliseconds to wait=u32 50) -> ()  [unwired: 1 out]
              }
              frame #2 {
                # "добавить RS"
                n493 = local write "Автомат"(TRUE ("Автомат")) -> ()
                n494 = Wait (ms)(milliseconds to wait=u32 3) -> ()  [unwired: 1 out]
              }
              frame #3 {
                n495 = local write "Start"(TRUE ("Start")) -> ()
              }
            }
          }
        }
        n496 = case shown="True" w868 {
          tunnel: w867 -> [_ _]
          frame False {
          }
          frame True {
            # "OFF"
            n497 = flat-sequence {
              frame #0 {
                w871 = FALSE ("PreCaptureIsDone")
                w870 = FALSE ("+6 ON")
                n498 = local write "+6 ON"(w870) -> ()
                n499 = local write "VDDD ON"(w870) -> ()
                n500 = local write "VDDA ON"(w870) -> ()
                n501 = local write "+0.5 ON"(w870) -> ()
                n502 = Wait (ms)(milliseconds to wait=u32 50) -> ()  [unwired: 1 out]
                n503 = local write "Frame Is Done"(w871) -> ()
                n504 = local write "PreCaptureIsDone"(w871) -> ()
                n505 = local write "Start"(w871) -> ()
                n506 = local write "Автомат"(w871) -> ()
              }
            }
          }
        }
      }
    }
    "Power OFF" <- w857
  }
  n507 = while {
    shift-right: [w888] -> _
    shift-left: FALSE ("+6 ON") -> [w887]
    tunnel: w3 -> [_]
    stop <- w885 stop-if-true
    # "Прошиваем АЦП через Configuration при включении питания +6"
    # "Цикл контроля АЦП"
    n508 = Wait (ms)(milliseconds to wait=u32 1) -> ()  [unwired: 1 out]
    n509 = local read "+6 ON"() -> (w888:bool)
    n510 = local read "SEL_warning"() -> (w881:bool)
    n511 = Greater?(x=w888, y=w887) -> (0:w882:bool)
    n512 = case shown="True" w882 {
      selector: w882 -> [w890 _]
      tunnel: [w890 w891] -> w883
      frame False {
      }
      frame True {
        n513 = while {
          tunnel: "ADC Rise Time" -> [w894]
          tunnel: [w893] -> w891
          i -> [w896]
          stop <- w893 stop-if-true
          n514 = To Long Integer(number=w894) -> (32bit integer=w895:i32)
          n515 = Wait (ms)(milliseconds to wait=u32 1) -> ()  [unwired: 1 out]
          n516 = Greater?(x=w896, y=w895) -> (0:w893:bool)
        }
      }
    }
    n517 = Not(x=w881) -> (.not. x?=w880:bool)
    n518 = Compound Arithmetic op=AND(w880, w883) -> (w884:bool)
    n519 = case shown="True" w884 {
      frame False {
      }
      frame True {
        n520 = flat-sequence {
          frame #0 {
            n521 = local write "ADC Register Map"(T4."Configuration" ("ADC Register Map")) -> ()
            "ADC Configuration" <- FALSE ("ADC Configuration")
          }
          frame #1 {
            n522 = local write "Прошить АЦП"(TRUE ("PreCapture")) -> ()
            n523 = Wait (ms)(milliseconds to wait=u32 5) -> ()  [unwired: 1 out]
          }
          frame #2 {
            n524 = while {
              stop <- w904 stop-if-true
              n525 = local read "STOP"() -> (w905:bool)
              n526 = local read "АЦП прошит!"() -> (w906:bool)
              n527 = Wait (ms)(milliseconds to wait=u32 1) -> ()  [unwired: 1 out]
              n528 = Or(x=w906, y=w905) -> (x .or. y?=w904:bool)
              n529 = local write "ADC Configuration"(w904) -> ()
            }
          }
          frame #3 {
            n530 = local write "Прошить АЦП"(FALSE ("Прошить АЦП")) -> ()
            n531 = Wait (ms)(milliseconds to wait=u32 5) -> ()  [unwired: 1 out]
          }
        }
      }
    }
    n532 = Less?(x=w888, y=w887) -> (x < y?=w889:bool)
    n533 = case shown="True" w889 {
      frame False {
      }
      frame True {
        n534 = local write "ADC Configuration"(FALSE ("ADC Configuration")) -> ()
        n535 = local write "АЦП прошит!"(FALSE ("ADC Configuration")) -> ()
      }
    }
    n536 = local read "STOP"() -> (w885:bool)
  }
  n537 = while {
    shift-right: [w912] -> _
    shift-left: FALSE ("POWER") -> [w914]
    tunnel: [w910] -> _
    tunnel: [w913] -> _
    tunnel: w3 -> [_]
    stop <- w910 stop-if-true
    n538 = Wait (ms)(milliseconds to wait="SEL Poll Time") -> ()  [unwired: 1 out]
    n539 = stacked-sequence {
      seq-local: [w915 _ _ _] -> [_ _ w1065 _]
      tunnel: w914 -> [w916 _ _ _]
      tunnel: [_ _ _ w1075] -> w910
      tunnel: [_ w1056 _ _] -> w913
      tunnel: [_ _ w1068 _] -> w912
      frame #0 {
        # "Детектирование SEL"
        n540 = local read "Питание"() -> (w915:bool)
        n541 = Greater?(x=w915, y=w916) -> (0:w917:bool)
        n542 = flat-sequence {
          tunnel: w917 -> [w922]
          tunnel: [w927] -> w921
          tunnel: [w926] -> w920
          tunnel: [w925] -> w919
          tunnel: [w924] -> w918
          tunnel: w921 -> [w944]
          tunnel: w920 -> [w943]
          tunnel: w919 -> [w942]
          tunnel: w918 -> [w941]
          frame #0 {
            n543 = case shown="True" w922 {
              frame False {
              }
              frame True {
                n544 = Wait (ms)(milliseconds to wait=u32 100) -> ()  [unwired: 1 out]
              }
            }
          }
          frame #1 {
            n545 = local read "VDDA_cur, A"() -> (w934:dbl)
            n546 = local read "VDDD_cur, A"() -> (w932:dbl)
            n547 = local read "+6_cur, A"() -> (w937:dbl)
            n548 = local read "+0.5_cur, A"() -> (w938:dbl)
            n549 = Greater Or Equal?(x=w934, y="VDDA_selcur, A") -> (x >= y?=w935:bool)
            n550 = Greater Or Equal?(x=w937, y="+6_selcur, A") -> (x >= y?=w925:bool)
            "+6_warning" <- w925
            n551 = Greater Or Equal?(x=w932, y="VDDD_selcur, A") -> (x >= y?=w931:bool)
            n552 = Greater Or Equal?(x=w938, y="+0.5_selcur, A") -> (x >= y?=w939:bool)
            n553 = Or(x="SIM_SEL", y=w935) -> (x .or. y?=w926:bool)
            "VDDD_warning" <- w926
            n554 = Or(x="SIM_SEL", y=w931) -> (x .or. y?=w927:bool)
            "VDDA_warning" <- w927
            n555 = Or(x="SIM_SEL", y=w939) -> (x .or. y?=w924:bool)
            "+0.5_warning" <- w924
            n556 = Compound Arithmetic op=OR(w927, w926, w925, w924) -> (→"SEL_warning":bool)
          }
          frame #2 {
            n557 = local read "SIM_SEL"() -> (w959:bool)
            n558 = Not(x=w959) -> (.not. x?=w945:bool)
            n559 = Select(t=TRUE, s="Считать SIM SEL", f=w945) -> (s? t:f=w950:bool)
            n560 = Select(t=TRUE, s="Считать SIM SEL", f=w945) -> (s? t:f=w947:bool)
            n561 = Select(t=TRUE, s="Считать SIM SEL", f=w945) -> (s? t:f=w957:bool)
            n562 = Select(t=TRUE, s="Считать SIM SEL", f=w945) -> (s? t:f=w954:bool)
            n563 = And(x=w943, y=w950) -> (x .and. y?=w952:bool)
            n564 = And(x=w941, y=w957) -> (x .and. y?=w956:bool)
            n565 = And(x=w942, y=w954) -> (x .and. y?=w953:bool)
            n566 = And(x=w944, y=w947) -> (x .and. y?=w949:bool)
            n567 = case shown="True" w949 {
              frame False {
                n568 = local read "VDDD_counter"() -> (w962:u32)
                n569 = Select(t=u32 0, s="VDDD_Clear_SEL", f=w962) -> (s? t:f=w960:u32)
                n570 = local write "VDDD_counter"(w960) -> ()
              }
              frame True {
                n571 = local read "VDDD_counter"() -> (w965:u32)
                n572 = Increment(x=w965) -> (x+1=→"VDDD_counter":u32)
              }
            }
            n573 = case shown="False" w952 {
              frame False {
                n574 = local read "VDDA_counter"() -> (w967:u32)
                n575 = Select(t=u32 0, s="VDDA_Clear_SEL", f=w967) -> (s? t:f=w969:u32)
                n576 = local write "VDDA_counter"(w969) -> ()
              }
              frame True {
                n577 = local read "VDDA_counter"() -> (w971:u32)
                n578 = Increment(x=w971) -> (x+1=→"VDDA_counter":u32)
              }
            }
            n579 = case shown="False" w953 {
              frame False {
                n580 = local read "+6_counter"() -> (w974:u32)
                n581 = Select(t=u32 0, s="+6_Clear_SEL", f=w974) -> (s? t:f=w972:u32)
                n582 = local write "+6_counter"(w972) -> ()
              }
              frame True {
                n583 = local read "+6_counter"() -> (w977:u32)
                n584 = Increment(x=w977) -> (x+1=→"+6_counter":u32)
              }
            }
            n585 = case shown="False" w956 {
              frame False {
                n586 = local read "+0.5_counter"() -> (w979:u32)
                n587 = Select(t=u32 0, s="+0.5_Clear_SEL", f=w979) -> (s? t:f=w981:u32)
                n588 = local write "+0.5_counter"(w981) -> ()
              }
              frame True {
                n589 = local read "+0.5_counter"() -> (w983:u32)
                n590 = Increment(x=w983) -> (x+1=→"+0.5_counter":u32)
              }
            }
          }
        }
      }
      frame #1 {
        w986 = "\t"
        w1011 = "\t"
        w1017 = "\t"
        w1018 = "\t"
        w1019 = "\t"
        w1020 = "\t"
        w987 = 0
        w1003 = 6
        # "Запись логов"
        n591 = local read "VDDA, V"() -> (w1000:dbl)
        n592 = local read "VDDA_cur, A"() -> (w999:dbl)
        n593 = local read "VDDD, V"() -> (w998:dbl)
        n594 = local read "VDDD_cur, A"() -> (w997:dbl)
        n595 = Multiply(x=w998, y=w997) -> (x*y=w1002:dbl)
        n596 = local read "Счетчик ОС"() -> (w991:u32)
        n597 = local read "Счетчик ФС"() -> (w990:u32)
        n598 = Multiply(x=w1000, y=w999) -> (x*y=w1001:dbl)
        n599 = local read "LED IR, V"() -> (w1012:dbl)
        n600 = local read "LED IR_cur, A"() -> (w1013:dbl)
        n601 = local read "VDDD_counter"() -> (w1054:u32)
        n602 = local read "VDDA_warning"() -> (w1055:bool)
        n603 = local read "VDDA_counter"() -> (w1053:u32)
        n604 = local read "VDDD_warning"() -> (w1052:bool)
        n605 = local read "+6, V"() -> (w1044:dbl)
        n606 = local read "+6_cur, A"() -> (w1046:dbl)
        n607 = local read "+6_counter"() -> (w1045:u32)
        n608 = local read "+6_warning"() -> (w1047:bool)
        n609 = local read "+0.5, V"() -> (w1043:dbl)
        n610 = local read "+0.5_cur, A"() -> (w1041:dbl)
        n611 = local read "+0.5_counter"() -> (w1042:u32)
        n612 = local read "+0.5_warning"() -> (w1040:bool)
        n613 = Add(x=w1001, y=w1002) -> (x+y=w994:dbl)
        n614 = Multiply(x=w994, y=1000.0) -> (x*y=w995:dbl)
        n615 = Number To Fractional String(number=w1043, precision (6)=w1003) -> (F-format string=w1025:string)  [unwired: 2 in]
        n616 = Number To Fractional String(number=w1041, precision (6)=w1003) -> (F-format string=w1024:string)  [unwired: 2 in]
        n617 = Number To Fractional String(number=w1042, precision (6)=w987) -> (F-format string=w1023:string)  [unwired: 2 in]
        n618 = Number To Fractional String(number=w1012, precision (6)=w1003) -> (F-format string=w1014:string)  [unwired: 2 in]
        n619 = Number To Fractional String(number=w1013, precision (6)=w1003) -> (F-format string=w1015:string)  [unwired: 2 in]
        n620 = Number To Fractional String(number=w1000, precision (6)=w1003) -> (F-format string=w1037:string)  [unwired: 2 in]
        n621 = Number To Fractional String(number=w999, precision (6)=w1003) -> (F-format string=w1036:string)  [unwired: 2 in]
        n622 = Number To Fractional String(number=w1054, precision (6)=w987) -> (F-format string=w1035:string)  [unwired: 2 in]
        n623 = Number To Fractional String(number=w998, precision (6)=w1003) -> (F-format string=w1033:string)  [unwired: 2 in]
        n624 = Number To Fractional String(number=w997, precision (6)=w1003) -> (F-format string=w1032:string)  [unwired: 2 in]
        n625 = Number To Fractional String(number=w1053, precision (6)=w987) -> (F-format string=w1031:string)  [unwired: 2 in]
        n626 = Number To Fractional String(number=w1044, precision (6)=w1003) -> (F-format string=w1029:string)  [unwired: 2 in]
        n627 = Number To Fractional String(number=w1046, precision (6)=w1003) -> (F-format string=w1028:string)  [unwired: 2 in]
        n628 = Number To Fractional String(number=w1045, precision (6)=w987) -> (F-format string=w1027:string)  [unwired: 2 in]
        n629 = Number To Fractional String(number=w995, precision (6)=i16 1) -> (F-format string=w1004:string)  [unwired: 2 in]
        n630 = Number To Fractional String(number=w991, precision (6)=w987) -> (F-format string=w989:string)  [unwired: 2 in]
        n631 = Number To Fractional String(number=w990, precision (6)=w987) -> (F-format string=w988:string)  [unwired: 2 in]
        n632 = Select(t="!!!_+0.5", s=w1040, f="") -> (s? t:f=w1022:string)
        n633 = Select(t="!!!_VDDD", s=w1055, f="") -> (s? t:f=w1034:string)
        n634 = Select(t="!!!_VDDA", s=w1052, f="") -> (s? t:f=w1030:string)
        n635 = Select(t="!!!_+6", s=w1047, f="") -> (s? t:f=w1026:string)
        n636 = Concatenate Strings(w1020, w1037, w1020, w1036, w1020, w1035, w1020, w1034) -> (w1010:string)
        n637 = Concatenate Strings(w1019, w1033, w1019, w1032, w1019, w1031, w1019, w1030) -> (w1009:string)
        n638 = Concatenate Strings(w1018, w1029, w1018, w1028, w1018, w1027, w1018, w1026) -> (w1008:string)
        n639 = Concatenate Strings(w1017, w1025, w1017, w1024, w1017, w1023, w1017, w1022) -> (w1007:string)
        n640 = Concatenate Strings(w1011, w1014, w1011, w1015) -> (w1006:string)
        n641 = Concatenate Strings("\t", w1004) -> (w996:string)
        "Power VDDD+VDDA, mW" <- w996
        n642 = Concatenate Strings(w986, w989, w986, w988) -> (w984:string)
        n643 = Get Date/Time In Seconds() -> (seconds since 1Jan1904=w1060:timestamp)
        n644 = Format Date/Time String(time format string (%c)="%H:%M:%S:%3u", seconds (now)=w1060) -> (date/time string=w1058:string)  [unwired: 1 in]
        n645 = local read "SEL output file refnum"() -> (w1016:refnum<file>)
        n646 = Concatenate Strings(w1058, w1010, w1009, w1008, w1007, w1006, w996, w984, "\r\n") -> (w1021:string)
        n647 = Format Into String(initial string=w1016, w1021) -> (resulting string=w1056:refnum<file>)  [unwired: 2 in, 1 out]
      }
      frame #2 {
        n648 = local read "VDDA_warning"() -> (w1067:bool)
        n649 = local read "VDDD_warning"() -> (w1066:bool)
        n650 = local read "+0.5_warning"() -> (w1064:bool)
        n651 = local read "+6_warning"() -> (w1062:bool)
        n652 = Compound Arithmetic op=OR(w1067, w1066, w1064, w1062) -> (w1063:bool)
        n653 = case shown="True" w1063 {
          tunnel: [w1069 w1070] -> w1068
          tunnel: w1065 -> [w1069 _]
          frame False {
          }
          frame True {
            n654 = flat-sequence {
              tunnel: [FALSE] -> w1070
              frame #0 {
                n655 = local write "Питание"(FALSE ("Power")) -> ()
              }
              frame #1 {
                n656 = Wait (ms)(milliseconds to wait=u32 100 ("Wait_parry, ms")) -> ()  [unwired: 1 out]
              }
              frame #2 {
                n657 = local write "Питание"(TRUE ("Power")) -> ()
              }
            }
          }
        }
      }
      frame #3 {
        n658 = local read "STOP"() -> (w1075:bool)
      }
    }
  }
  n659 = while {
    shift-right: ["Capture"] -> _
    shift-left: FALSE ("Кадр готов") -> [w1090]
    tunnel: w9 -> [w1084]
    tunnel: w3 -> [_]
    tunnel: [w1091] -> w8
    shift-right: ["Loop Capture"] -> _
    shift-left: FALSE ("Loop Capture") -> [w1081]
    tunnel: w4 -> [w1078]
    stop <- w1098 stop-if-true
    n660 = local read "ADC Configuration"() -> (w1092:bool)
    n661 = local read "Frame Is Done"() -> (w1088:bool)
    n662 = local read "SEL_warning"() -> (w1095:bool)
    n663 = local read "PreCaptureIsDone"() -> (w1096:bool)
    n664 = local read "ОС"() -> (w1080:bool)
    n665 = local read "ФС"() -> (w1077:bool)
    n666 = Greater?(x="Capture", y=w1090) -> (0:w1099:bool)
    n667 = Less?(x="Loop Capture", y=w1081) -> (x < y?=w1083:bool)
    n668 = Or(x="Loop Capture", y=w1099) -> (x .or. y?=w1097:bool)
    n669 = Not(x=w1080) -> (.not. x?=w1079:bool)
    n670 = Not(x=w1077) -> (.not. x?=w1076:bool)
    n671 = Not(x=w1095) -> (.not. x?=w1094:bool)
    n672 = And(x=w1088, y=w1083) -> (x .and. y?=w1085:bool)
    n673 = Less?(x="Capture", y=w1090) -> (x < y?=w1086:bool)
    n674 = Or(x=w1086, y=w1085) -> (x .or. y?=w1087:bool)
    n675 = Compound Arithmetic op=AND(w1094, w1096, w1097, w1092, w1079, w1076) -> (w1100:bool)
    n676 = case shown="True" w1087 {
      tunnel: w1084 -> [_ w1101]
      frame False {
      }
      frame True {
        n677 = xnode "Read/Write Control"("FPGA VI Reference In"=w1101, "CSTop"=FALSE, "CSBot"=FALSE) -> ()  [unwired: 1 in, 2 out]
      }
    }
    n678 = case shown="True" w1100 {
      tunnel: [w1105 w1109] -> w1098
      tunnel: w1084 -> [w1104 w1108]
      tunnel: [w1104 w1107] -> w1091
      tunnel: w1078 -> [_ w1106]
      frame False {
        n679 = local read "STOP"() -> (w1105:bool)
      }
      frame True {
        n680 = stacked-sequence {
          tunnel: [_ _ _ _ _ _ w1378] -> w1109
          tunnel: w1108 -> [w1114 w1116 _ w1220 _ _ w1377]
          tunnel: [_ _ _ _ _ _ w1377] -> w1107
          tunnel: w1106 -> [_ _ _ _ _ _ w1376]
          frame #0 {
            n681 = xnode "Read/Write Control"("FPGA VI Reference In"=w1114, "CSTop"=TRUE, "CSBot"=TRUE) -> ()  [unwired: 1 in, 2 out]
            n682 = Wait (ms)(milliseconds to wait=u32 3) -> ()  [unwired: 1 out]
            "Frame Is Done" <- FALSE ("Frame Is Done")
          }
          frame #1 {
            n683 = case shown="True" "Top" {
              tunnel: w1116 -> [_ w1117]
              frame False {
              }
              frame True {
                # "Принимаем кадр с Top"
                n684 = stacked-sequence {
                  tunnel: w1117 -> [w1118 w1136 w1172 _]
                  frame #0 {
                    n685 = flat-sequence {
                      frame #0 {
                        n686 = local write "ADC Register Map"(T4."MUX" ("ADC Register Map")) -> ()
                        n687 = local write "Какой канал?"("TopVIN") -> ()
                        n688 = Wait (ms)(milliseconds to wait=u32 5) -> ()  [unwired: 1 out]
                      }
                      frame #1 {
                        n689 = local write "Прошить АЦП"(TRUE ("Прошить АЦП")) -> ()
                        n690 = Wait (ms)(milliseconds to wait=u32 5) -> ()  [unwired: 1 out]
                      }
                      frame #2 {
                        n691 = while {
                          stop <- w1132 stop-if-true
                          n692 = local read "АЦП прошит!"() -> (w1131:bool)
                          n693 = local read "STOP"() -> (w1130:bool)
                          n694 = Wait (ms)(milliseconds to wait=u32 1) -> ()  [unwired: 1 out]
                          n695 = Or(x=w1131, y=w1130) -> (x .or. y?=w1132:bool)
                        }
                      }
                      frame #3 {
                        n696 = Wait (ms)(milliseconds to wait=u32 5) -> ()  [unwired: 1 out]
                        n697 = local write "Прошить АЦП"(FALSE ("Прошить АЦП")) -> ()
                      }
                    }
                    n698 = xnode "Invoke Method"("FPGA VI Reference In"=w1118, "Number of Elements"=u32 0, "Timeout (ms)"=0) -> ("FPGA VI Reference Out"=w1124:refnum<k20>, "error out"=w1123:errorcluster, "Elements Remaining"=w1120:u32)  [unwired: 1 in, 1 out]
                    n699 = xnode "Invoke Method"("FPGA VI Reference In"=w1124, "error in"=w1123, "Number of Elements"=w1120, "Timeout (ms)"=0) -> ()  [unwired: 4 out]
                  }
                  frame #1 {
                    n700 = for {
                      N: 3 -> [_]
                      tunnel: w1136 -> [w1142]
                      i -> [w1143]
                      n701 = flat-sequence {
                        tunnel: w1143 -> [w1149]
                        tunnel: w1142 -> [w1144]
                        tunnel: [w1145] -> w1141
                        tunnel: [w1144] -> w1140
                        tunnel: w1141 -> [w1152]
                        tunnel: w1140 -> [w1154]
                        tunnel: [w1151] -> w1139
                        tunnel: w1139 -> [w1155]
                        tunnel: [w1155] -> w1138
                        tunnel: w1138 -> [w1163]
                        frame #0 {
                          n702 = Wait (ms)(milliseconds to wait=u32 5) -> ()  [unwired: 1 out]
                          n703 = Add(x=w1149, y=2) -> (x+y=w1147:i32)
                          n704 = local write "Этап прошивки"(w1147) -> ()
                          n705 = Equal?(x=w1147, y=4) -> (x = y?=w1145:bool)
                        }
                        frame #1 {
                          n706 = xnode "Read/Write Control"("FPGA VI Reference In"=w1154, "FrameToFIFO"=w1152) -> ("FPGA VI Reference Out"=w1151:refnum<k20>)  [unwired: 1 in, 1 out]
                          n707 = Wait (ms)(milliseconds to wait=u32 1) -> ()  [unwired: 1 out]
                        }
                        frame #2 {
                          n708 = local read "Этап прошивки"() -> (w1161:T2)
                          n709 = local write "Firmware"(TRUE ("Firmware")) -> ()
                          n710 = Equal?(x=w1161, y=T2."Hold") -> (x = y?=w1159:bool)
                          n711 = Select(t="Frame Exposure, ms", s=w1159, f=u32 5 ("milliseconds to wait")) -> (s? t:f=w1157:u32)
                          n712 = Wait (ms)(milliseconds to wait=w1157) -> ()  [unwired: 1 out]
                        }
                        frame #3 {
                          n713 = while {
                            tunnel: w1163 -> [w1165]
                            stop <- w1167 stop-if-true
                            n714 = local read "FirmwareIsDone"() -> (w1169:bool)
                            n715 = local read "STOP"() -> (w1168:bool)
                            n716 = Wait (ms)(milliseconds to wait=u32 1) -> ()  [unwired: 1 out]
                            n717 = xnode "Read/Write Control"("FPGA VI Reference In"=w1165, "FrameToFIFO"=FALSE) -> ()  [unwired: 1 in, 2 out]
                            n718 = Or(x=w1169, y=w1168) -> (x .or. y?=w1167:bool)
                          }
                        }
                      }
                    }
                  }
                  frame #2 {
                    n719 = flat-sequence {
                      tunnel: [w1175] -> w1171
                      tunnel: w1172 -> [w1174]
                      tunnel: w1171 -> [w1187]
                      tunnel: [w1186] -> w1170
                      tunnel: [w1191] -> w1173
                      tunnel: w1170 -> [w1190]
                      tunnel: w1173 -> [w1201]
                      tunnel: [w1202] -> _
                      frame #0 {
                        n720 = while {
                          tunnel: [w1185] -> w1175
                          tunnel: w1174 -> [w1177]
                          i -> [w1178]
                          stop <- w1183 stop-if-true
                          n721 = xnode "Read/Write Control"("FPGA VI Reference In"=w1177) -> ("FPGA VI Reference Out"=w1185:refnum<k20>, "FIFOIsDone"=w1181:bool)  [unwired: 1 in, 1 out]
                          n722 = Wait (ms)(milliseconds to wait=u32 2) -> ()  [unwired: 1 out]
                          n723 = local read "STOP"() -> (w1182:bool)
                          n724 = To Unsigned Long Integer(number=w1178) -> (unsigned 32bit integer=w1180:u32)
                          "FIFOTime" <- w1180
                          n725 = Greater?(x=w1180, y="WatchDogFIFOTime") -> (0:w1176:bool)
                          n726 = Compound Arithmetic op=OR(w1182, w1181, w1176) -> (w1183:bool)
                        }
                      }
                      frame #1 {
                        n727 = xnode "Read/Write Control"("FPGA VI Reference In"=w1187, "ResetFIFO"=TRUE ("ReseSendData")) -> ("FPGA VI Reference Out"=w1186:refnum<k20>)  [unwired: 1 in, 1 out]
                        n728 = Wait (ms)(milliseconds to wait=u32 1) -> ()  [unwired: 1 out]
                      }
                      frame #2 {
                        n729 = while {
                          tunnel: w1190 -> [w1192]
                          tunnel: [w1196] -> w1191
                          stop <- w1195 stop-if-true
                          n730 = xnode "Read/Write Control"("FPGA VI Reference In"=w1192) -> ("FPGA VI Reference Out"=w1198:refnum<k20>, "FIFOIsDone"=w1193:bool)  [unwired: 1 in, 1 out]
                          n731 = local read "STOP"() -> (w1197:bool)
                          n732 = Wait (ms)(milliseconds to wait=u32 1) -> ()  [unwired: 1 out]
                          n733 = Not(x=w1193) -> (.not. x?=w1194:bool)
                          n734 = Or(x=w1194, y=w1197) -> (x .or. y?=w1195:bool)
                          n735 = xnode "Read/Write Control"("FPGA VI Reference In"=w1198, "ResetFIFO"=w1193) -> ("FPGA VI Reference Out"=w1196:refnum<k20>)  [unwired: 1 in, 1 out]
                        }
                      }
                      frame #3 {
                        n736 = xnode "Invoke Method"("FPGA VI Reference In"=w1201, "Number of Elements"=u32 0, "Timeout (ms)"=0) -> ("FPGA VI Reference Out"=w1208:refnum<k20>, "error out"=w1207:errorcluster, "Elements Remaining"=w1206:u32)  [unwired: 1 in, 1 out]
                        n737 = xnode "Invoke Method"("FPGA VI Reference In"=w1208, "error in"=w1207, "Number of Elements"=w1206, "Timeout (ms)"=0) -> ("FPGA VI Reference Out"=w1202:refnum<k20>, "Data"=→"FrameDataFromTop":u8[])  [unwired: 2 out]
                        n738 = Wait (ms)(milliseconds to wait=u32 5) -> ()  [unwired: 1 out]
                      }
                    }
                  }
                  frame #3 {
                    n739 = flat-sequence {
                      frame #0 {
                        n740 = local write "Этап прошивки"(T2."Sample End" ("Этап прошивки")) -> ()
                        n741 = Wait (ms)(milliseconds to wait=u32 5) -> ()  [unwired: 1 out]
                      }
                      frame #1 {
                        n742 = local write "Firmware"(TRUE ("Firmware")) -> ()
                        n743 = Wait (ms)(milliseconds to wait=u32 5) -> ()  [unwired: 1 out]
                      }
                      frame #2 {
                        n744 = while {
                          stop <- w1215 stop-if-true
                          n745 = local read "FirmwareIsDone"() -> (w1217:bool)
                          n746 = local read "STOP"() -> (w1216:bool)
                          n747 = Wait (ms)(milliseconds to wait=u32 1) -> ()  [unwired: 1 out]
                          n748 = Or(x=w1217, y=w1216) -> (x .or. y?=w1215:bool)
                        }
                      }
                    }
                  }
                }
              }
            }
          }
          frame #2 {
            n749 = Wait (ms)(milliseconds to wait="Delay Between Top&Bot") -> ()  [unwired: 1 out]
          }
          frame #3 {
            n750 = case shown="True" "Bot" {
              tunnel: w1220 -> [_ w1221]
              frame False {
              }
              frame True {
                # "Принимаем кадр с Bot"
                n751 = stacked-sequence {
                  tunnel: w1221 -> [w1222 w1240 w1276 _]
                  frame #0 {
                    n752 = flat-sequence {
                      frame #0 {
                        n753 = local write "ADC Register Map"(T4."MUX" ("ADC Register Map")) -> ()
                        n754 = local write "Какой канал?"("Bot VIN") -> ()
                        n755 = Wait (ms)(milliseconds to wait=u32 5) -> ()  [unwired: 1 out]
                      }
                      frame #1 {
                        n756 = local write "Прошить АЦП"(TRUE ("Прошить АЦП")) -> ()
                        n757 = Wait (ms)(milliseconds to wait=u32 5) -> ()  [unwired: 1 out]
                      }
                      frame #2 {
                        n758 = while {
                          stop <- w1236 stop-if-true
                          n759 = local read "АЦП прошит!"() -> (w1235:bool)
                          n760 = local read "STOP"() -> (w1234:bool)
                          n761 = Wait (ms)(milliseconds to wait=u32 1) -> ()  [unwired: 1 out]
                          n762 = Or(x=w1235, y=w1234) -> (x .or. y?=w1236:bool)
                        }
                      }
                      frame #3 {
                        n763 = local write "Прошить АЦП"(FALSE ("Прошить АЦП")) -> ()
                        n764 = Wait (ms)(milliseconds to wait=u32 5) -> ()  [unwired: 1 out]
                      }
                    }
                    n765 = xnode "Invoke Method"("FPGA VI Reference In"=w1222, "Number of Elements"=u32 0, "Timeout (ms)"=0) -> ("FPGA VI Reference Out"=w1226:refnum<k20>, "error out"=w1225:errorcluster, "Elements Remaining"=w1224:u32)  [unwired: 1 in, 1 out]
                    n766 = xnode "Invoke Method"("FPGA VI Reference In"=w1226, "error in"=w1225, "Number of Elements"=w1224, "Timeout (ms)"=0) -> ()  [unwired: 4 out]
                  }
                  frame #1 {
                    n767 = for {
                      N: 3 -> [_]
                      tunnel: w1240 -> [w1246]
                      i -> [w1247]
                      n768 = flat-sequence {
                        tunnel: w1247 -> [w1253]
                        tunnel: w1246 -> [w1249]
                        tunnel: [w1249] -> w1245
                        tunnel: [w1248] -> w1244
                        tunnel: w1245 -> [w1258]
                        tunnel: w1244 -> [w1257]
                        tunnel: [w1255] -> w1243
                        tunnel: w1243 -> [w1259]
                        tunnel: [w1259] -> w1242
                        tunnel: w1242 -> [w1267]
                        frame #0 {
                          n769 = Add(x=w1253, y=2) -> (x+y=w1251:i32)
                          n770 = local write "Этап прошивки"(w1251) -> ()
                          n771 = Equal?(x=w1251, y=4) -> (x = y?=w1248:bool)
                          n772 = Wait (ms)(milliseconds to wait=u32 5) -> ()  [unwired: 1 out]
                        }
                        frame #1 {
                          n773 = xnode "Read/Write Control"("FPGA VI Reference In"=w1258, "FrameToFIFO"=w1257) -> ("FPGA VI Reference Out"=w1255:refnum<k20>)  [unwired: 1 in, 1 out]
                          n774 = Wait (ms)(milliseconds to wait=u32 1) -> ()  [unwired: 1 out]
                        }
                        frame #2 {
                          n775 = local read "Этап прошивки"() -> (w1265:T2)
                          n776 = Equal?(x=w1265, y=T2."Hold") -> (x = y?=w1263:bool)
                          n777 = local write "Firmware"(TRUE ("Firmware")) -> ()
                          n778 = local read "Frame Exposure, ms"() -> (w1260:u32)
                          n779 = Select(t=w1260, s=w1263, f=u32 5 ("milliseconds to wait")) -> (s? t:f=w1262:u32)
                          n780 = Wait (ms)(milliseconds to wait=w1262) -> ()  [unwired: 1 out]
                        }
                        frame #3 {
                          n781 = while {
                            tunnel: w1267 -> [w1268]
                            stop <- w1271 stop-if-true
                            n782 = local read "FirmwareIsDone"() -> (w1273:bool)
                            n783 = local read "STOP"() -> (w1272:bool)
                            n784 = Wait (ms)(milliseconds to wait=u32 1) -> ()  [unwired: 1 out]
                            n785 = xnode "Read/Write Control"("FPGA VI Reference In"=w1268, "FrameToFIFO"=FALSE) -> ()  [unwired: 1 in, 2 out]
                            n786 = Or(x=w1273, y=w1272) -> (x .or. y?=w1271:bool)
                          }
                        }
                      }
                    }
                  }
                  frame #2 {
                    n787 = flat-sequence {
                      tunnel: [w1279] -> w1275
                      tunnel: w1276 -> [w1278]
                      tunnel: w1275 -> [w1291]
                      tunnel: [w1290] -> w1274
                      tunnel: [w1295] -> w1277
                      tunnel: w1274 -> [w1294]
                      tunnel: w1277 -> [w1305]
                      frame #0 {
                        n788 = while {
                          tunnel: [w1289] -> w1279
                          tunnel: w1278 -> [w1281]
                          i -> [w1284]
                          stop <- w1287 stop-if-true
                          n789 = xnode "Read/Write Control"("FPGA VI Reference In"=w1281) -> ("FPGA VI Reference Out"=w1289:refnum<k20>, "FIFOIsDone"=w1285:bool)  [unwired: 1 in, 1 out]
                          n790 = Wait (ms)(milliseconds to wait=u32 2) -> ()  [unwired: 1 out]
                          n791 = local read "WatchDogFIFOTime"() -> (w1283:u32)
                          n792 = To Unsigned Long Integer(number=w1284) -> (unsigned 32bit integer=w1282:u32)
                          n793 = local read "STOP"() -> (w1286:bool)
                          n794 = Greater?(x=w1282, y=w1283) -> (0:w1280:bool)
                          n795 = local write "FIFOTime"(w1282) -> ()
                          n796 = Compound Arithmetic op=OR(w1286, w1285, w1280) -> (w1287:bool)
                        }
                      }
                      frame #1 {
                        n797 = xnode "Read/Write Control"("FPGA VI Reference In"=w1291, "ResetFIFO"=TRUE ("ReseSendData")) -> ("FPGA VI Reference Out"=w1290:refnum<k20>)  [unwired: 1 in, 1 out]
                        n798 = Wait (ms)(milliseconds to wait=u32 1) -> ()  [unwired: 1 out]
                      }
                      frame #2 {
                        n799 = while {
                          tunnel: w1294 -> [w1296]
                          tunnel: [w1300] -> w1295
                          stop <- w1298 stop-if-true
                          n800 = xnode "Read/Write Control"("FPGA VI Reference In"=w1296) -> ("FPGA VI Reference Out"=w1302:refnum<k20>, "FIFOIsDone"=w1297:bool)  [unwired: 1 in, 1 out]
                          n801 = local read "STOP"() -> (w1301:bool)
                          n802 = Wait (ms)(milliseconds to wait=u32 1) -> ()  [unwired: 1 out]
                          n803 = Not(x=w1297) -> (.not. x?=w1299:bool)
                          n804 = Or(x=w1299, y=w1301) -> (x .or. y?=w1298:bool)
                          n805 = xnode "Read/Write Control"("FPGA VI Reference In"=w1296) -> ()  [unwired: 2 in, 2 out]
                          n806 = xnode "Read/Write Control"("FPGA VI Reference In"=w1302, "ResetFIFO"=w1297) -> ("FPGA VI Reference Out"=w1300:refnum<k20>)  [unwired: 1 in, 1 out]
                        }
                      }
                      frame #3 {
                        n807 = xnode "Invoke Method"("FPGA VI Reference In"=w1305, "Number of Elements"=u32 0, "Timeout (ms)"=0) -> ("FPGA VI Reference Out"=w1311:refnum<k20>, "error out"=w1310:errorcluster, "Elements Remaining"=w1309:u32)  [unwired: 1 in, 1 out]
                        n808 = xnode "Invoke Method"("FPGA VI Reference In"=w1311, "error in"=w1310, "Number of Elements"=w1309, "Timeout (ms)"=0) -> ("Data"=→"FrameDataFromBot":u8[])  [unwired: 3 out]
                        n809 = Wait (ms)(milliseconds to wait=u32 5) -> ()  [unwired: 1 out]
                      }
                    }
                  }
                  frame #3 {
                    n810 = flat-sequence {
                      frame #0 {
                        n811 = local write "Этап прошивки"(T2."Sample End" ("Этап прошивки")) -> ()
                        n812 = Wait (ms)(milliseconds to wait=u32 5) -> ()  [unwired: 1 out]
                      }
                      frame #1 {
                        n813 = local write "Firmware"(TRUE ("Firmware")) -> ()
                        n814 = Wait (ms)(milliseconds to wait=u32 5) -> ()  [unwired: 1 out]
                      }
                      frame #2 {
                        n815 = while {
                          stop <- w1318 stop-if-true
                          n816 = local read "FirmwareIsDone"() -> (w1320:bool)
                          n817 = local read "STOP"() -> (w1319:bool)
                          n818 = Wait (ms)(milliseconds to wait=u32 1) -> ()  [unwired: 1 out]
                          n819 = Or(x=w1320, y=w1319) -> (x .or. y?=w1318:bool)
                        }
                      }
                    }
                  }
                }
              }
            }
          }
          frame #4 {
            # "Выгружаем массив FIFO в массивы Top и Bot"
            n820 = local read "1032 pixels"() -> (w1323:u16)
            n821 = To Long Integer(number=w1323) -> (32bit integer=w1321:i32)
            n822 = for {
              N: w1321 -> [_]
              shift-right: [w1348] -> _
              shift-left: 0 -> [w1346]
              i -> [w1350]
              n823 = local read "FrameDataFromTop"() -> (w1360:u8[])
              n824 = Increment(x=w1346) -> (x+1=w1345:i32)
              n825 = Index Array(array=w1360, index=w1345) -> (element=w1359:u8)
              n826 = Index Array(array=w1360, index=w1346) -> (element=w1358:u8)
              n827 = Number To Boolean Array(number=w1359) -> (Boolean array=w1344:bool[])
              n828 = Number To Boolean Array(number=w1358) -> (Boolean array=w1343:bool[])
              n829 = local read "Top Pixel"() -> (w1357:bool[])
              n830 = Replace Array Subset(array=w1357, new element #1=w1344, index #1=0 ("index"), new element #2=w1343, index #2=8 ("index")) -> (w1347:bool[])
              "Top Pixel" <- w1347
              n831 = Boolean Array To Number(Boolean array=w1347) -> (number=w1354:u32)
              n832 = To Unsigned Word Integer(number=w1354) -> (unsigned 16bit integer=w1353:u16)
              n833 = local read "LineOfTop"() -> (w1351:u16[])
              n834 = Replace Array Subset(array=w1351, new element=w1353, index=w1350) -> (→"LineOfTop":u16[])
              n835 = Add(x=w1346, y=2) -> (x+y=w1348:i32)
            }
            n836 = for {
              N: w1321 -> [_]
              shift-right: [w1329] -> _
              shift-left: 0 -> [w1325]
              i -> [w1331]
              n837 = local read "FrameDataFromBot"() -> (w1342:u8[])
              n838 = Increment(x=w1325) -> (x+1=w1326:i32)
              n839 = Index Array(array=w1342, index=w1326) -> (element=w1341:u8)
              n840 = Index Array(array=w1342, index=w1325) -> (element=w1340:u8)
              n841 = Number To Boolean Array(number=w1341) -> (Boolean array=w1338:bool[])
              n842 = Number To Boolean Array(number=w1340) -> (Boolean array=w1337:bool[])
              n843 = local read "Bot Pixel"() -> (w1339:bool[])
              n844 = Replace Array Subset(array=w1339, new element #1=w1338, index #1=0 ("index"), new element #2=w1337, index #2=8 ("index")) -> (w1327:bool[])
              "Bot Pixel" <- w1327
              n845 = Boolean Array To Number(Boolean array=w1327) -> (number=w1334:u32)
              n846 = To Unsigned Word Integer(number=w1334) -> (unsigned 16bit integer=w1333:u16)
              n847 = local read "LineOfBot"() -> (w1332:u16[])
              n848 = Replace Array Subset(array=w1332, new element=w1333, index=w1331) -> (→"LineOfBot":u16[])
              n849 = Add(x=w1325, y=2) -> (x+y=w1329:i32)
            }
          }
          frame #5 {
            n850 = local read "1032 pixels"() -> (w1362:u16)
            n851 = To Long Integer(number=w1362) -> (32bit integer=w1361:i32)
            n852 = for {
              N: w1361 -> [_]
              shift-right: [w1370] -> _
              shift-left: 0 -> [w1366]
              i -> [w1364]
              n853 = Increment(x=w1366) -> (x+1=w1369:i32)
              n854 = local read "LineOfTop"() -> (w1373:u16[])
              n855 = local read "LineOfBot"() -> (w1374:u16[])
              n856 = Index Array(array=w1373, index=w1364) -> (element=w1372:u16)
              n857 = Index Array(array=w1374, index=w1364) -> (element=w1371:u16)
              n858 = local read "Full Line"() -> (w1368:u16[])
              n859 = Replace Array Subset(array=w1368, new element #1=w1372, index #1=w1366, new element #2=w1371, index #2=w1369) -> (→"Full Line":u16[])
              n860 = Add(x=2 ("y"), y=w1366) -> (x+y=w1370:i32)
            }
          }
          frame #6 {
            # "Выгружаем кадр"
            n861 = case shown="\"Top / Bot\", Default" "Capture Format" {
              tunnel: w1376 -> [w1379 w1404]
              frame "Top / Bot", Default {
                n862 = flat-sequence {
                  tunnel: w1379 -> [w1383]
                  frame #0 {
                    w1381 = 24 ("x")
                    n863 = Multiply(x=2, y=w1381) -> (x*y=w1380:i32)
                    n864 = for {
                      N: w1380 -> [_]
                      shift-right: [w1392] -> _
                      shift-left: 0 -> [w1393]
                      tunnel: [w1399] -> w1385 mode=indexing
                      tunnel: w1381 -> [w1395]
                      i -> [w1396]
                      w1398 = 43 ("length")
                      n865 = Less?(x=w1395, y=w1396) -> (x < y?=w1397:bool)
                      n866 = case shown="False" w1397 {
                        tunnel: [w1400 w1401] -> w1390
                        frame False {
                          n867 = local read "LineOfTop"() -> (w1400:u16[])
                        }
                        frame True {
                          n868 = local read "LineOfBot"() -> (w1401:u16[])
                        }
                      }
                      n869 = local read "1032 pixels"() -> (w1389:u16)
                      n870 = Add(x=w1398, y=w1393) -> (x+y=w1387:i32)
                      n871 = Array Subset(array=w1390, index=w1393, length=w1398) -> (w1399:u16[])
                      n872 = To Long Integer(number=w1389) -> (32bit integer=w1388:i32)
                      n873 = Equal?(x=w1388, y=w1387) -> (x = y?=w1394:bool)
                      n874 = Select(t=0, s=w1394, f=w1387) -> (s? t:f=w1392:i32)
                    }
                    n875 = call "IMAQ ArrayToImage"("Image Pixels (U16)"=w1385, "Image"=w1383) -> ("Image Out"=→"Image":T3)  [unwired: 8 in, 1 out]
                  }
                  frame #1 {
                    n876 = local write "Frame Is Done"(TRUE ("Кадр готов")) -> ()
                    n877 = Wait (ms)(milliseconds to wait=u32 5) -> ()  [unwired: 1 out]
                  }
                }
              }
              frame "Top & Bot" {
                n878 = flat-sequence {
                  tunnel: w1404 -> [w1408]
                  frame #0 {
                    n879 = local read "Full Line"() -> (w1405:u16[])
                    n880 = for {
                      N: 48 ("x") -> [_]
                      shift-right: [w1412] -> _
                      shift-left: 0 -> [w1413]
                      tunnel: [w1415] -> w1410 mode=indexing
                      tunnel: w1405 -> [w1411]
                      w1414 = 43 ("length")
                      n881 = Add(x=w1414, y=w1413) -> (x+y=w1412:i32)
                      n882 = Array Subset(array=w1411, index=w1413, length=w1414) -> (w1415:u16[])
                    }
                    n883 = call "IMAQ ArrayToImage"("Image Pixels (U16)"=w1410, "Image"=w1408) -> ("Image Out"=w1407:T3)  [unwired: 8 in, 1 out]
                    n884 = local write "Image"(w1407) -> ()
                  }
                  frame #1 {
                    n885 = local write "Frame Is Done"(TRUE ("Кадр готов")) -> ()
                    n886 = Wait (ms)(milliseconds to wait=u32 5) -> ()  [unwired: 1 out]
                  }
                }
              }
            }
            n887 = local read "STOP"() -> (w1378:bool)
            n888 = case shown="False" w1378 {
              frame False {
              }
              frame True {
                n889 = local write "Loop Capture"(FALSE ("Loop Capture")) -> ()
              }
            }
          }
        }
      }
    }
    n890 = Wait (ms)(milliseconds to wait="Frame Poll Time") -> ()  [unwired: 1 out]
  }
  n891 = call <instrlib>:"niDCPower Close.vi"("instrument handle"=w12) -> ()  [unwired: 10 in, 1 out]
  n892 = call <instrlib>:"niDCPower Close.vi"("instrument handle"=w11) -> ()  [unwired: 10 in, 1 out]
  n893 = while {
    tunnel: w3 -> [_]
    stop <- w1420 stop-if-true
    n894 = Wait (ms)(milliseconds to wait=u32 200) -> ()  [unwired: 1 out]
    n895 = case shown="True" "Очистить ОС" {
      frame False {
      }
      frame True {
        n896 = local write "Очистить ОС"(FALSE ("Очистить ОС")) -> ()
        n897 = local write "Счетчик ОС"(u32 0 ("t")) -> ()
      }
    }
    n898 = case shown="True" "Плюс ОС" {
      frame False {
      }
      frame True {
        n899 = local read "Счетчик ОС"() -> (w1444:u32)
        n900 = local write "Плюс ОС"(FALSE ("Плюс ОС")) -> ()
        n901 = Add(x=w1444, y=u32 1 ("t")) -> (x+y=w1442:u32)
        n902 = local write "Счетчик ОС"(w1442) -> ()
      }
    }
    n903 = case shown="True" "Минус ОС" {
      frame False {
      }
      frame True {
        n904 = local read "Счетчик ОС"() -> (w1440:u32)
        n905 = local write "Минус ОС"(FALSE ("Минус ОС")) -> ()
        n906 = Subtract(x=w1440, y=u32 1 ("t")) -> (x-y=w1438:u32)
        n907 = local write "Счетчик ОС"(w1438) -> ()
      }
    }
    n908 = case shown="True" "Очистить ФС" {
      frame False {
      }
      frame True {
        n909 = local write "Очистить ФС"(FALSE ("Очистить ФС")) -> ()
        n910 = local write "Счетчик ФС"(u32 0 ("t")) -> ()
      }
    }
    n911 = case shown="False" "Плюс ФС" {
      frame False {
      }
      frame True {
        n912 = local read "Счетчик ФС"() -> (w1434:u32)
        n913 = local write "Плюс ФС"(FALSE ("Плюс ФС")) -> ()
        n914 = Add(x=w1434, y=u32 1 ("t")) -> (x+y=w1432:u32)
        n915 = local write "Счетчик ФС"(w1432) -> ()
      }
    }
    n916 = case shown="True" "Минус ФС" {
      frame False {
      }
      frame True {
        n917 = local read "Счетчик ФС"() -> (w1430:u32)
        n918 = local write "Минус ФС"(FALSE ("Минус ФС")) -> ()
        n919 = Subtract(x=w1430, y=u32 1 ("t")) -> (x-y=w1428:u32)
        n920 = local write "Счетчик ФС"(w1428) -> ()
      }
    }
    n921 = local read "STOP"() -> (w1420:bool)
  }
  n922 = while {
    tunnel: w3 -> [_]
    shift-right: [w1451] -> _
    shift-left: FALSE ("ФС") -> [w1450]
    stop <- w1453 stop-if-true
    # "При ФС отключаем питание и через некоторое время возвращаем его в предыдущее состояние (чтобы через ФС не включалась схема, когда она выключена)\nЕсли принимался кадр, то ждем завершения Capture / Loop Capture"
    # "Контроль ФС"
    n923 = local read "SEL_warning"() -> (w1447:bool)
    n924 = Wait (ms)(milliseconds to wait=u32 1) -> ()  [unwired: 1 out]
    n925 = Not(x=w1447) -> (.not. x?=w1448:bool)
    n926 = And(x="ФС", y=w1448) -> (x .and. y?=w1454:bool)
    n927 = case shown="True" w1454 {
      tunnel: w1450 -> [_ w1455]
      frame False {
      }
      frame True {
        n928 = stacked-sequence {
          tunnel: w1455 -> [_ _ w1465]
          frame #0 {
            n929 = local read "Loop Capture"() -> (w1457:bool)
            n930 = local read "Capture"() -> (w1458:bool)
            n931 = Or(x=w1458, y=w1457) -> (x .or. y?=w1456:bool)
            n932 = case shown="True" w1456 {
              frame False {
              }
              frame True {
                n933 = while {
                  stop <- w1460 stop-if-true
                  n934 = local read "STOP"() -> (w1461:bool)
                  n935 = local read "Frame Is Done"() -> (w1462:bool)
                  n936 = Or(x=w1462, y=w1461) -> (x .or. y?=w1460:bool)
                  n937 = Wait (ms)(milliseconds to wait=u32 1) -> ()  [unwired: 1 out]
                }
              }
            }
          }
          frame #1 {
            n938 = local write "Питание"(FALSE ("Питание")) -> ()
            n939 = Wait (ms)(milliseconds to wait=u32 100) -> ()  [unwired: 1 out]
          }
          frame #2 {
            n940 = local read "Счетчик ФС"() -> (w1467:u32)
            n941 = local write "Питание"(w1465) -> ()
            n942 = Increment(x=w1467) -> (x+1=→"Счетчик ФС":u32)
            n943 = local write "ФС"(FALSE ("ФС")) -> ()
          }
        }
      }
    }
    n944 = local read "STOP"() -> (w1453:bool)
    n945 = local read "Питание"() -> (w1451:bool)
  }
  n946 = while {
    tunnel: w9 -> [w1508]
    tunnel: w3 -> [_]
    stop <- w1507 stop-if-true
    # "Инициализация служебных переменных Target"
    n947 = Wait (ms)(milliseconds to wait=u32 1) -> ()  [unwired: 1 out]
    n948 = xnode "Read/Write Control"("FPGA VI Reference In"=w1508, "NumberOfAddFIFO"="NumberOfAddFIFO", "R MCLK = 2"="R MCLK = 2", "R ADCCLK = 5"="R ADCCLK = 5", "1032 pixels"="1032 pixels", "Command CS"="Command CS", "Data CSTop"="Data CSTop", "Data CSBot"="Data CSBot", "Command Reset"="Command Reset", "Data Reset"="Data Reset", "Command Hold"="Command Hold", "Data Hold"="Data Hold", "Command Sample Start"="Command Sample Start", "Data Sample Start"="Data Sample Start", "Command Sample End"="Command Sample End", "Data Sample End"="Data Sample End", "Counter R CLK = 2"="Counter R CLK = 2", "Rising CLK_1 = 0"="Rising CLK_1 = 0", "Falling CLK_1 = 1"="Falling CLK_1 = 1", "Rising CLK_2 = 1"="Rising CLK_2 = 1", "Falling CLK_2 = 2"="Falling CLK_2 = 2", "Rising CLK_5 = 2"="Rising CLK_5 = 2", "Falling CLK_5 = 2"="Falling CLK_5 = 2", "Rising CLK_3 = 1"="Rising CLK_3 = 1", "Falling CLK_4 = 3"="Falling CLK_4 = 3", "Counter R&F CLK_1 = 7"="Counter R&F CLK_1 = 7", "Rising CLK_6 = 2"="Rising CLK_6 = 2", "Falling CLK_6 = 2"="Falling CLK_6 = 2", "Rising CLK_7 = 1"="Rising CLK_7 = 1", "Falling CLK_7 = 1"="Falling CLK_7 = 1", "Counter R&F CLK_2 = 4"="Counter R&F CLK_2 = 4", "Rising CLK_4 = 2"="Rising CLK_4 = 2", "Falling CLK_3 = 1"="Falling CLK_3 = 1", "Supply Select"="Supply Select") -> ("Data"=→"Data":u8[], "Command"=→"Command":u8[], "ArraySize"=→"ArraySize":u8, "FIFOCounter"=→"FIFOCounter":u16)  [unwired: 1 in, 2 out]
    n949 = local read "STOP"() -> (w1507:bool)
  }
  n950 = xnode "Read/Write Control"("FPGA VI Reference In"=w8, "Stop_FPGA"=TRUE) -> ("FPGA VI Reference Out"=w6:refnum<k20>)  [unwired: 1 in, 1 out]
  n951 = xnode "Close FPGA VI Reference"("FPGA VI Reference In"=w6) -> ()  [unwired: 1 in, 1 out]
  n952 = Close File(refnum=w15) -> ()  [unwired: 1 in, 2 out]
  n953 = call <instrlib>:"niDMM Close.vi"("instrument handle"=w14) -> ()  [unwired: 10 in, 1 out]
